vi "ChannelAutomatorR.vi"() -> ()   [LabVIEW 2020]
uses:
  <vilib>/Platform/TimedLoop/XDataNode/timing_clust.ctl
  <vilib>/Platform/TimedLoop/XDataNode/nitl_modes.ctl
  <vilib>/Platform/TimedLoop/XDataNode/wakeup.ctl
  bbe0dff6-800f-412b-80fa-b33fe90fb9f3.vi
  <vilib>/DAQmx/read.llb/DAQmx Read (Analog 1D Wfm NChan NSamp).vi
  <vilib>/DAQmx/write.llb/DAQmx Write (Analog 1D Wfm NChan NSamp).vi
  <vilib>/DAQmx/create/channels.llb/DAQmx Create Channel (AI-Voltage-Basic).vi
  <vilib>/httpClient/POSTBuffer.vi
  <vilib>/DAQmx/miscellaneous.llb/DAQmx Fill In Error Info.vi
  <vilib>/DAQmx/configure/timing.llb/DAQmx Timing (Sample Clock).vi
  <vilib>/DAQmx/create/channels.llb/DAQmx Create Channel (AO-Voltage-Basic).vi
  <vilib>/Comparison/Less/Less Functor/Less Functor.lvclass
  <vilib>/Platform/TimedLoop/XDataNode/XDataNode.xnode
  <resource>/objmgr/daqmx.rc
  <vilib>/httpClient/LabVIEWHTTPClient.lvlib
  <vilib>/wsapi/NI_WebServices.lvlib
  <vilib>/measure/NI_MABase.lvlib
  <vilib>/Platform/TimedLoop/XDataNode/XDNodeRunTimeDep.lvlib
  <vilib>/ptbypt/NI_PtbyPt.lvlib
panel:
  out "stds":dbl[](array[numeric])
  out "Means":dbl[](array[numeric])
  out "frequency":dbl=20.0
  out "fileCreateTime":timestamp
  out "headers":string
  out "timed out?":bool
  out "# elements in queue":i32
  out "body 2":string
  out "error out 3":errorcluster
  out "error out 2":errorcluster
  out "body":string
  in  "Tab Control 2":enum32{"RT Monitor", "IV Monitor"}(tab)
  out "Channel 4":waveform(dbl)[](graph)
  out "Channel 3":waveform(dbl)[](graph)
  out "Channel 2":waveform(dbl)[](graph)
  out "XY Graph":cluster{"Y":dbl[], "Y":dbl[]}[](graph)
  out "XY Graph 2":cluster{"Y":dbl[], "Y":dbl[]}[](graph)
  out "XY Graph 3":cluster{"Y":dbl[], "Y":dbl[]}[](graph)
  out "XY Graph 4":cluster{"Y":dbl[], "Y":dbl[]}[](graph)
  out "output path":path
  out "FilenameValid":bool
  out "ParameterNames":string[](array[string])=["Wafer", "Notes", "Experiment Name", "Buffer", "Bias Voltage", "Reference Electrode", "Chip", "Analyte"]
  out "ParameterValues":string[](array[string])
  out "RT Monitoring 2":bool
  out "error out":errorcluster
  out "StopProgram":bool
  out "FileOpen":bool
  out "tdms file out":refnum<k34>
  in  "Tab Control":enum32{"Data View", "Settings"}(tab)
  in  "TraceTime":dbl=30.0
  in  "IV Monitoring":bool
  in  "RT Monitoring":bool
  out "Recording":bool
  in  "Record":bool
  in  "Reference Voltage (mV)":string
  in  "Bias Voltage (mV)":string
  in  "Experiment Name":string
  in  "Wafer, Chip":string
  in  "Notes":string
  in  "Buffer":string
  in  "Analyte":string
  in  "DB48":bool
  in  "DB37":bool
  in  "Device Banks":bool
  in  "DB26":bool
  in  "Channels":string="N2,N6,E2,E6,S2,S6,W2,W6"
  out "Warnings":string="Wrong number of Channel Names!"
  out "Monitoring":bool
  in  "DataDirectory":path=path "C:/DempBot_Data"
  in  "Queue Size":i32=100
  in  "Channel 9":tag="Dev1/ai0"
  in  "Channel 10":tag="Dev1/ai2"
  in  "Channel 11":tag="Dev1/ai3"
  in  "Channel 12":tag="Dev1/ai4"
  in  "Channel 13":tag="Dev1/ai5"
  in  "Channel 14":tag="Dev1/ai6"
  in  "Channel 15":tag="Dev1/ai7"
  in  "Channel 16":tag="Dev1/ai8"
  in  "Sampling Rate:":dbl=5000.0
  in  "Recorded Channels":i32=8
  in  "No. of Samples / Loop":i64=1000
  in  "Gain (V/nA)":dbl=-0.45
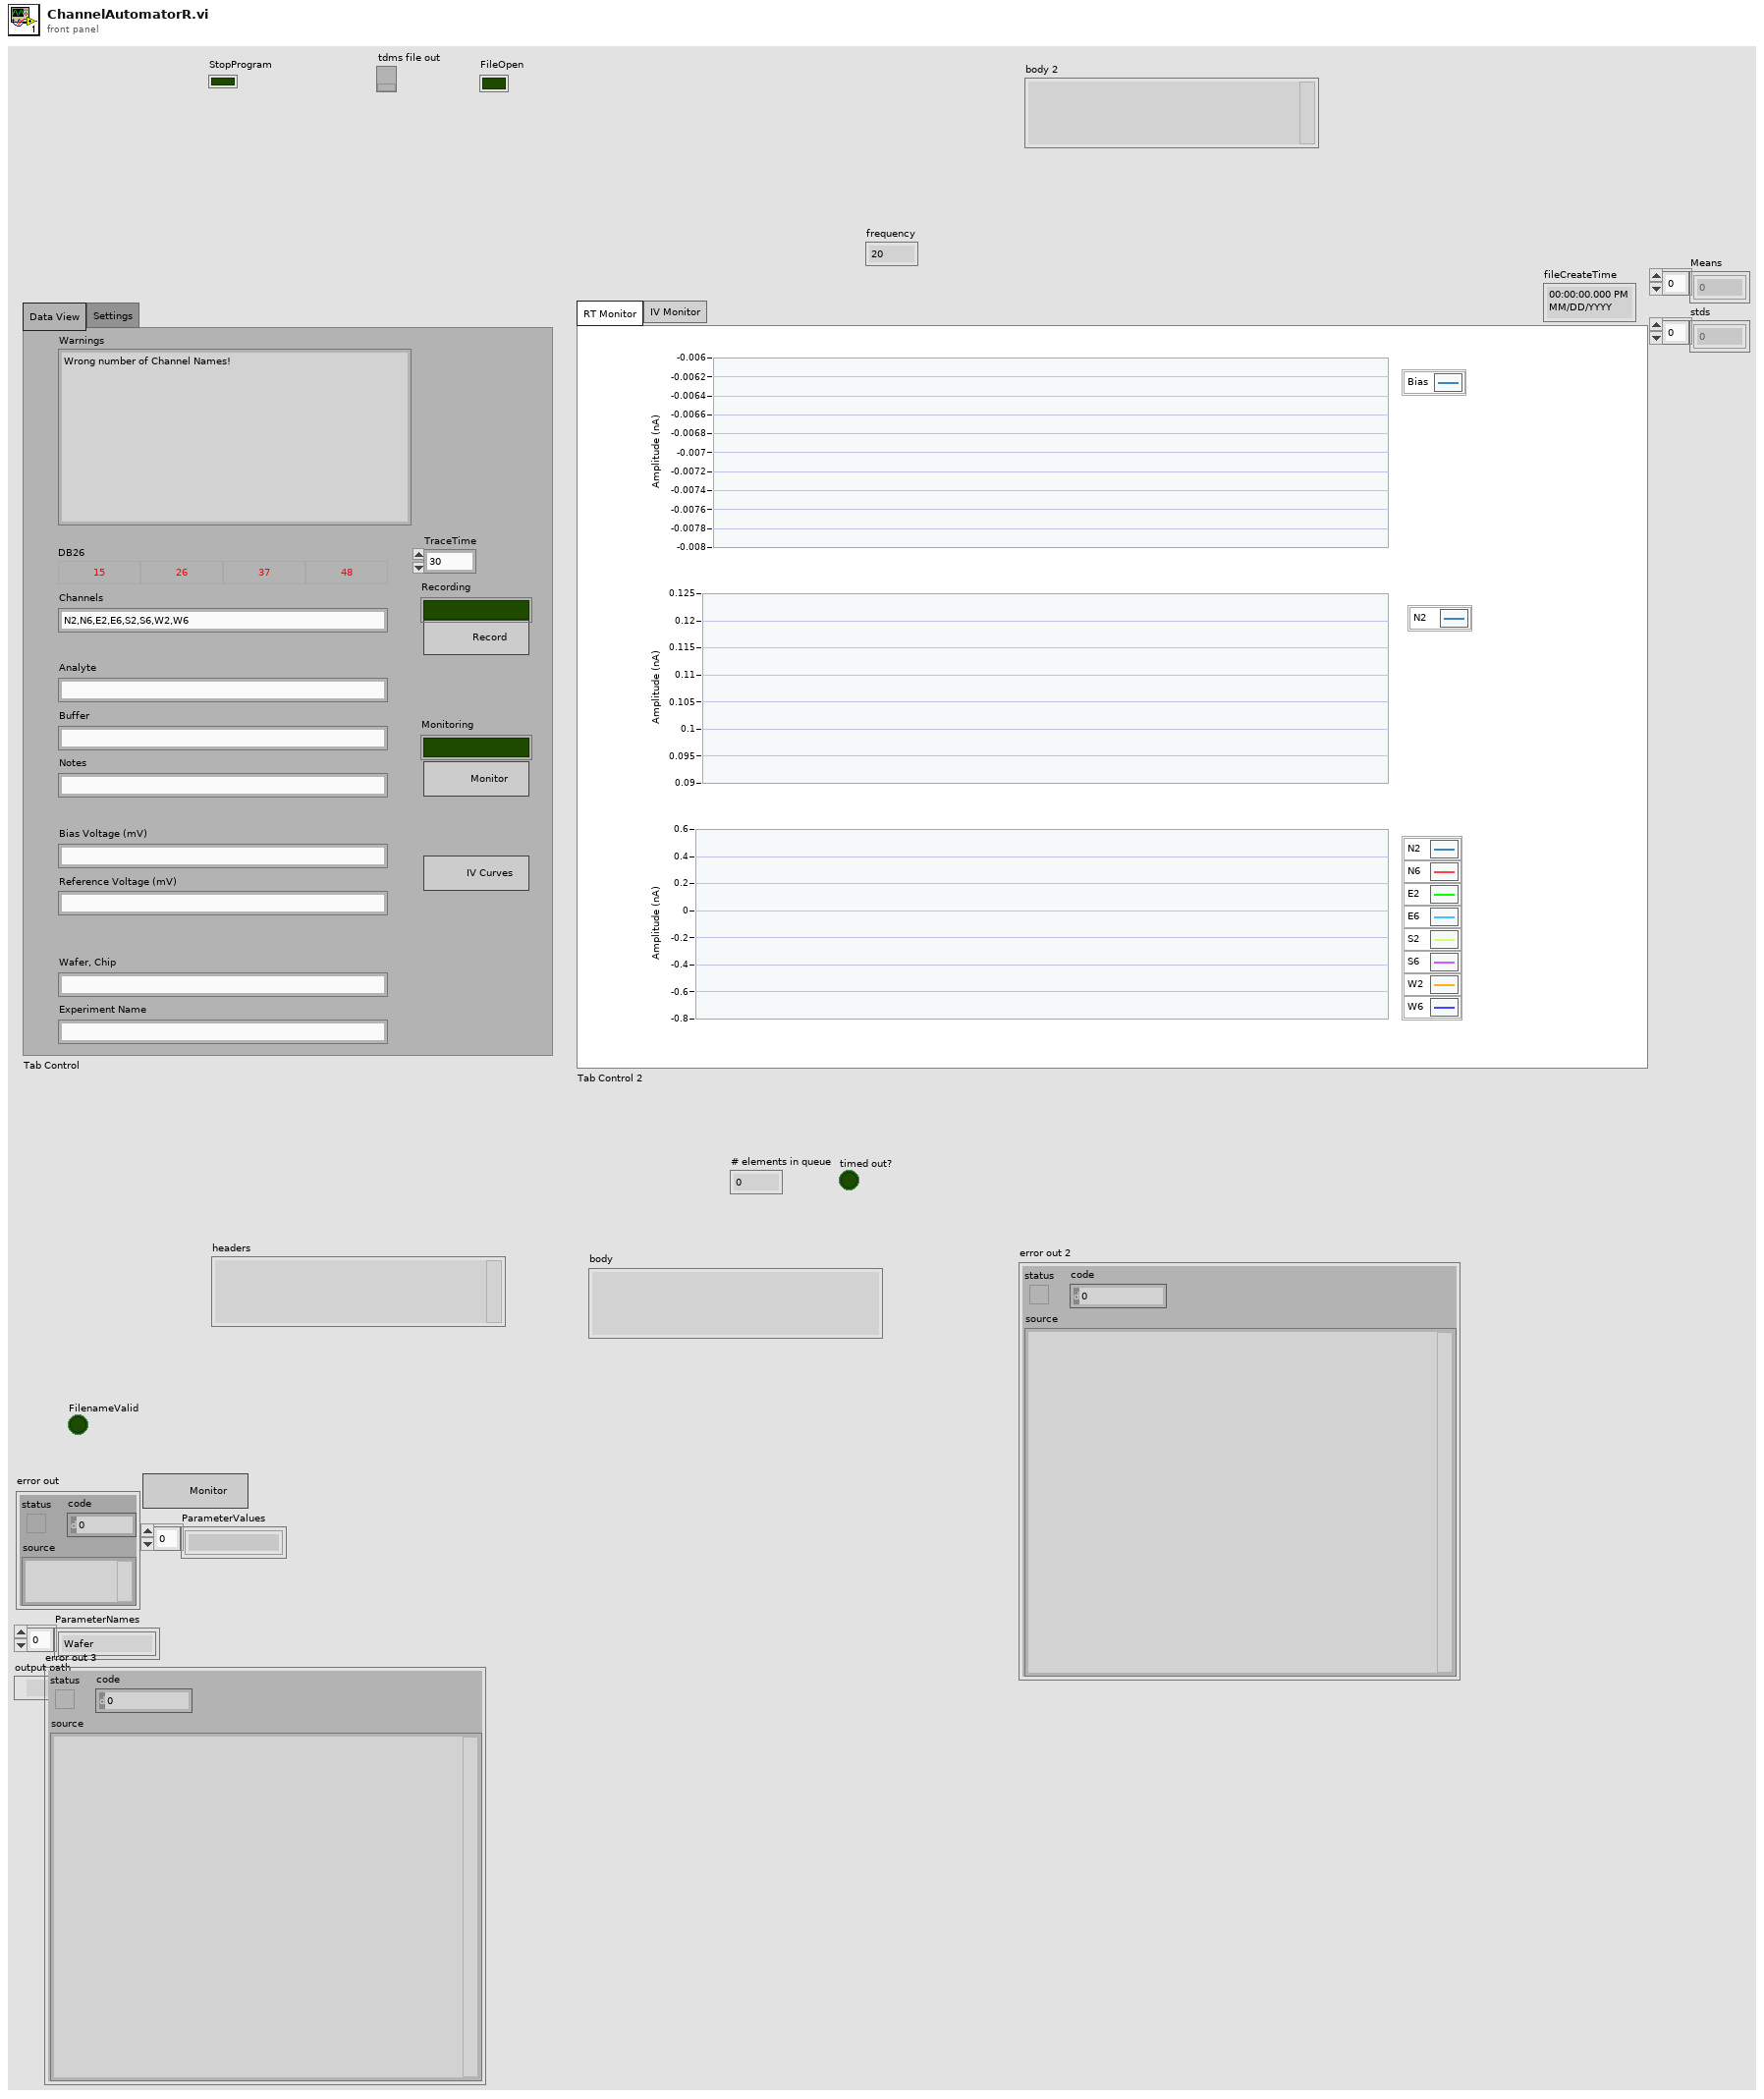
[diagram p1: front panel]
types:
  T1 = cluster{"command":string, "machine":string, "payload":string}
  T2 = typedef "LabVIEWHTTPClient.lvlib/ClientHandle.ctl" = refnum<k1>
  T3 = enum16{"open", "open or create", "create or replace", "create", "open (read-only)"}
  T4 = typedef "XDNodeRunTimeDep.lvlib/timing_clust.ctl" = cluster{"Expected End [f-1]":u64, "Actual End [f-1]":u64, "Finished Late? [f-1]":bool, "Expected End [i-1]":u64, "Actual End [i-1]":u64, "Finished Late? [i-1]":bool, "Expected Start [i]":u64, "Actual Start [i]":u64, "Expected Start [f]":u64, "Actual Start [f]":u64, "Source Name":string, "Structure Name":string, "Period":i64, "Deadline":i64, "Offset":i64, "Start":i64, "Priority":i32, "Timeout":i32, "Mode":T5, "Wakeup Reason":T6, "Error":errorcluster, "Source Type":string, "Secondary Source Type":string, "Global End Time":u64, "Global Start Time":u64, "Frame Duration":u64, "Iteration Duration":u64, "Assigned CPU":i32, "I/O Scan Engine Mode":u32}
  T5 = typedef "XDNodeRunTimeDep.lvlib/nitl_modes.ctl" = enum32{"No Change", "Process missed periods, maintain original phase", "Discard missed periods, maintain original phase", "Process missed periods, ignore original phase", "Discard missed periods, ignore original phase"}
  T6 = typedef "XDNodeRunTimeDep.lvlib/wakeup.ctl" = enum32{"Normal", "Aborted", "Asynchronous wakeup", "Timing source error", "Timed loop error", "Timeout"}
  T7 = enum16{"Sine Wave", "Triangle Wave", "Square Wave", "Sawtooth Wave"}
  T8 = cluster{"channelNames":string[], "dt":dbl, "traces":sgl[][], "dataType":string, "means":dbl[], "stds":dbl[]}
  T9 = cluster{"channels":string, "analyte":string, "notes":string, "buffer":string, "experiment":string, "waferChip":string}
  T10 = cluster{"duration":dbl, "bias":dbl, "frequency":dbl}
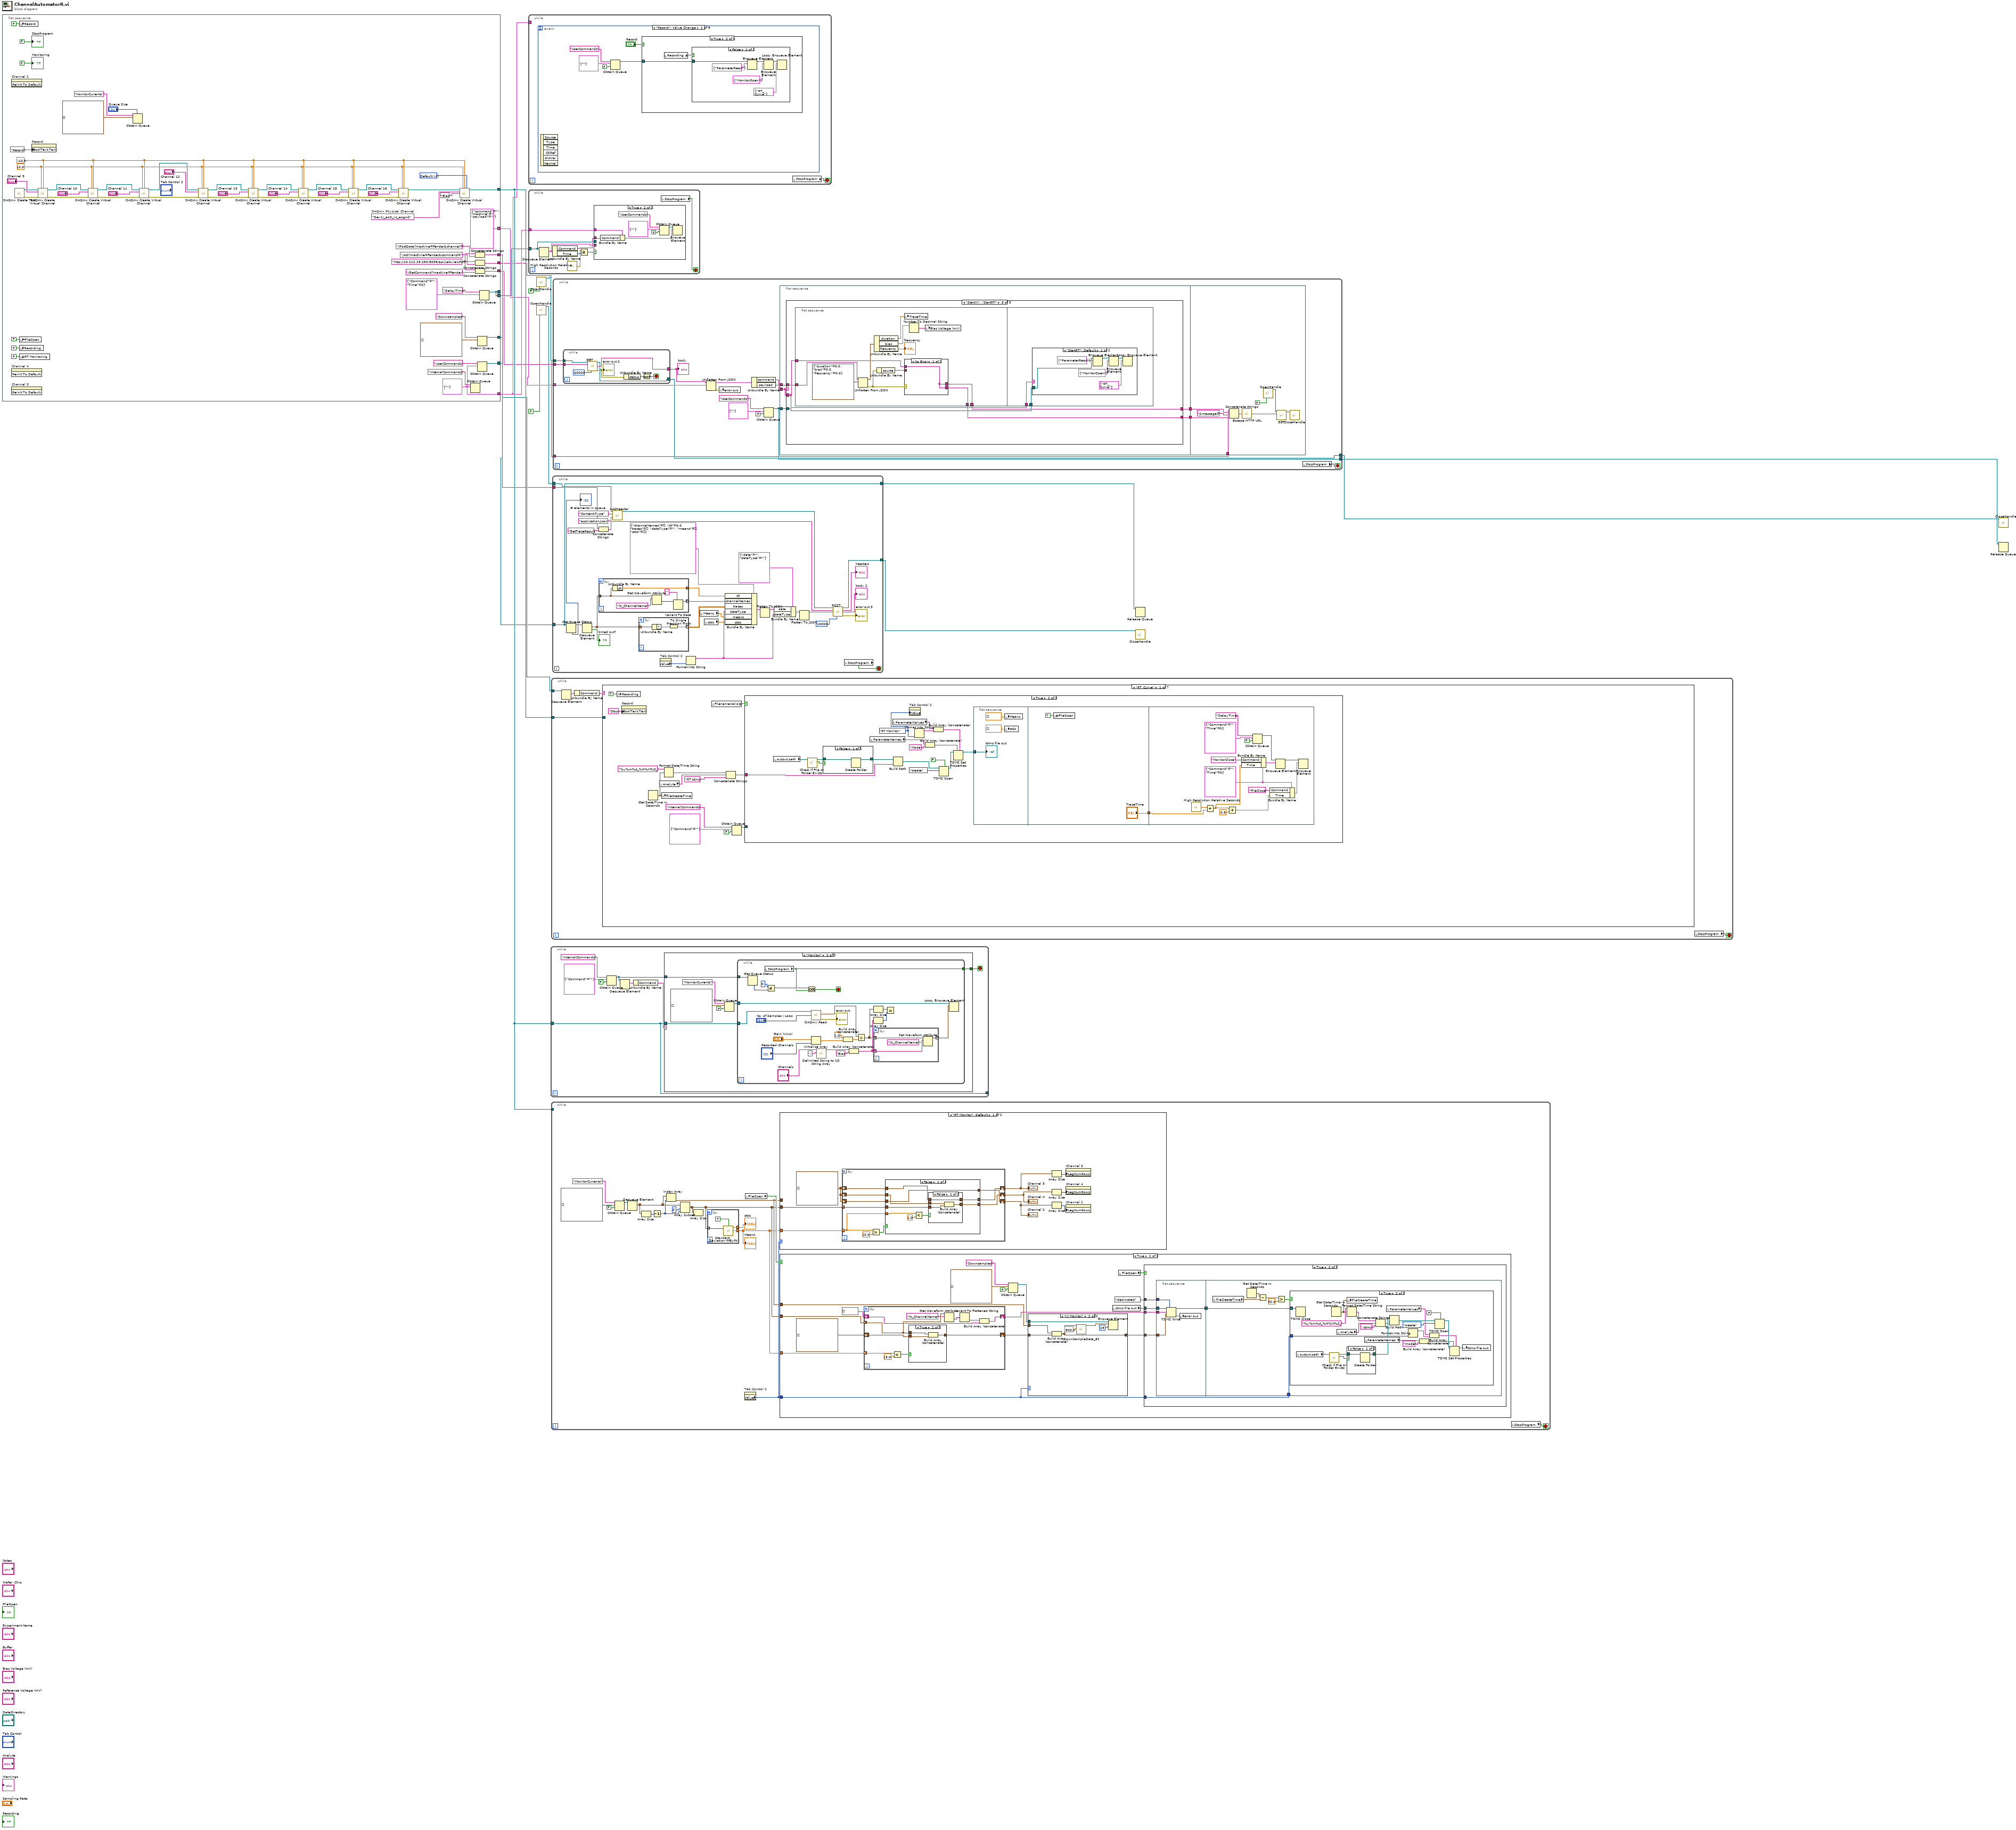
[diagram p0: block diagram]
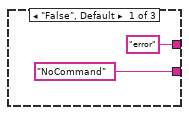
[diagram p2: hidden frame]
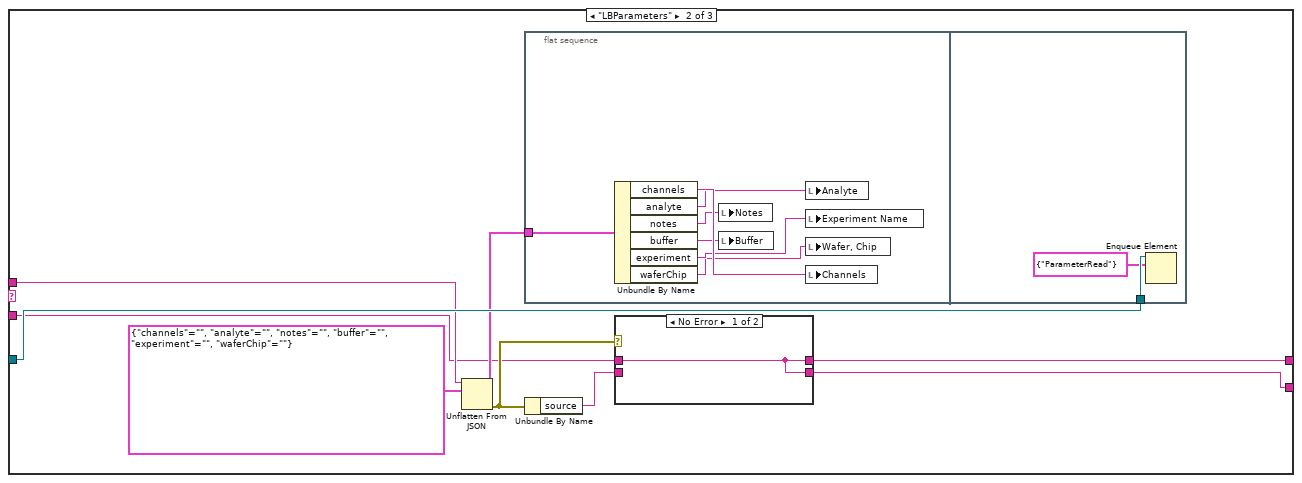
[diagram p3: hidden frame]
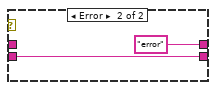
[diagram p4: hidden frame]
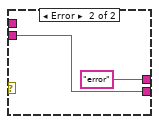
[diagram p5: hidden frame]
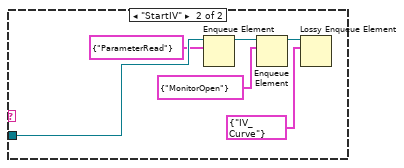
[diagram p6: hidden frame]
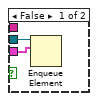
[diagram p7: hidden frame]
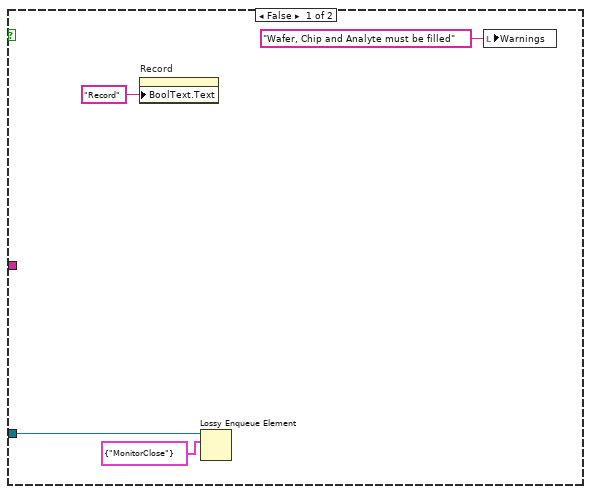
[diagram p8: hidden frame]
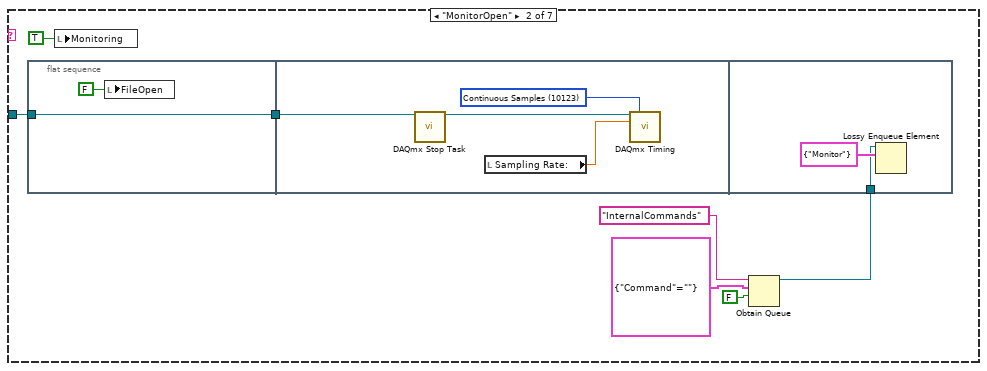
[diagram p10: hidden frame]
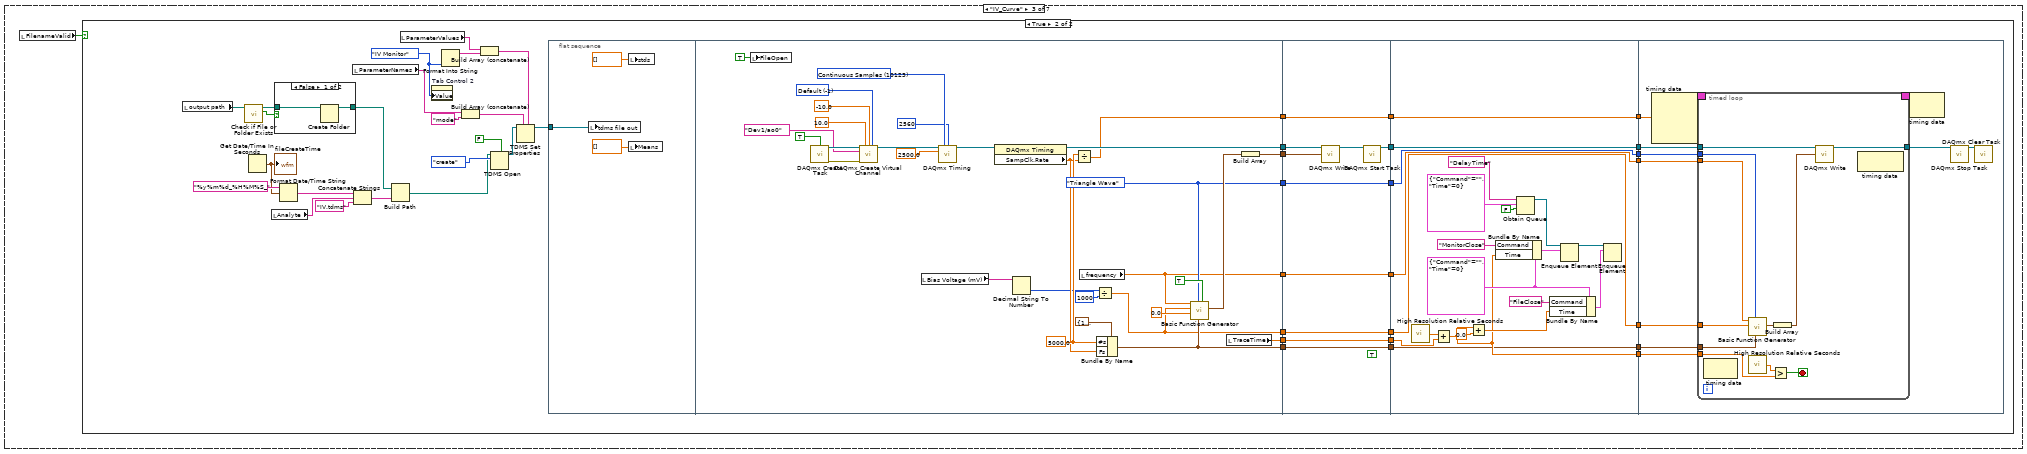
[diagram p11: hidden frame]
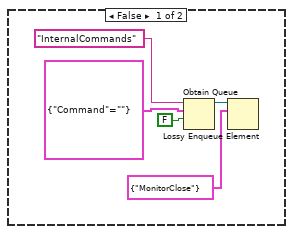
[diagram p12: hidden frame]
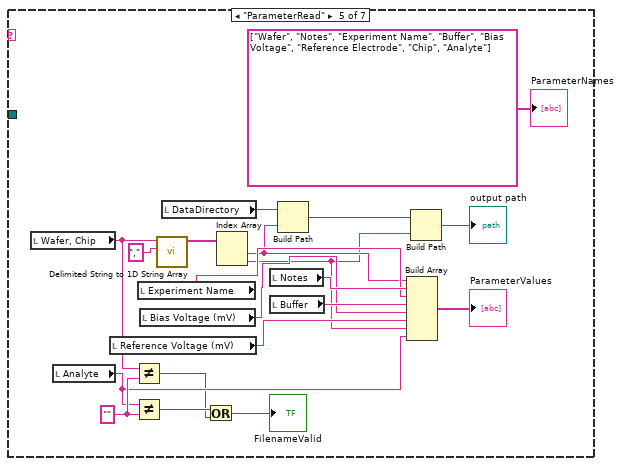
[diagram p15: hidden frame]
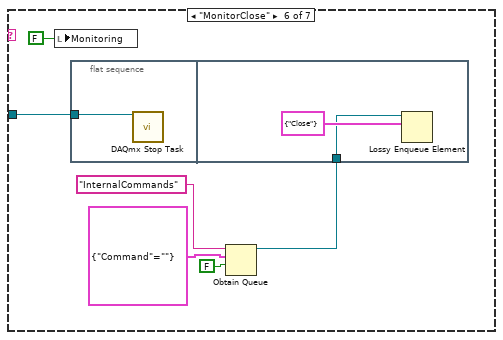
[diagram p16: hidden frame]
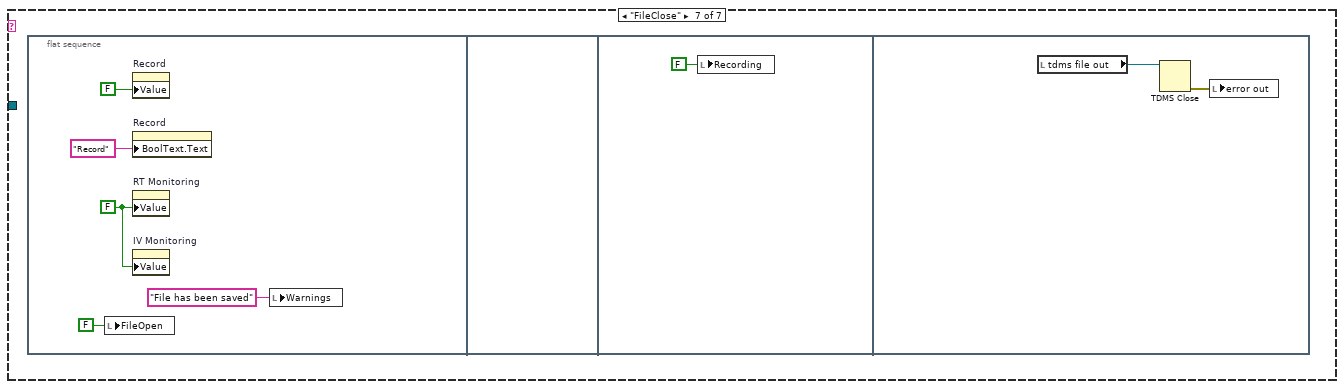
[diagram p17: hidden frame]
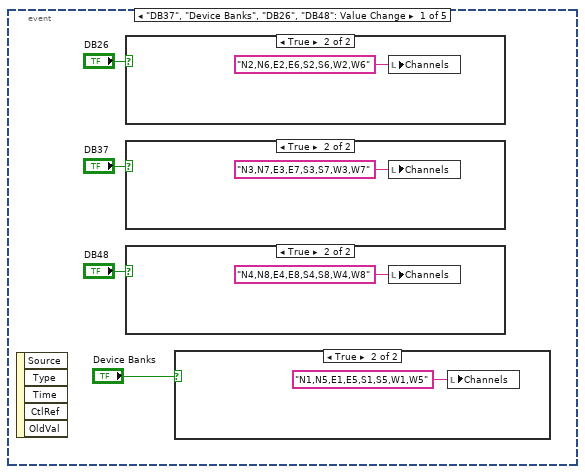
[diagram p18: hidden frame]
diagram:
  n1 = flat-sequence {
    tunnel: [w35] -> w17
    tunnel: [w40] -> w15
    tunnel: [w30] -> w16
    tunnel: [w34] -> w14
    tunnel: [w30] -> _
    tunnel: [T1 {"command"="", "machine"="", "payload"=""}] -> w13
    tunnel: [w28] -> w12
    tunnel: [w23] -> w9
    tunnel: [w22] -> w8
    tunnel: [w24] -> w1
    frame #0 {
      w20 = -1 items=["Default"=-1, "RSE"=10083, "NRSE"=10078, "Differential"=10106, "Pseudodifferential"=12529] ("input terminal configuration")
      w21 = "http://10.212.29.250:8038/api/LabviewPoll"
      w42 = tag "Dev1/_ao0_vs_aognd"  # DAQmx Physical Channel
      w34 = cluster{"Command":string} {"Command"=""}
      w19 = -10.0 ("minimum value")
      w18 = 10.0 ("maximum value")
      n2 = invoke on="Channel 2" class="WFChart (strict)" method="Reinit To Default"() -> ()  [unwired: 3 in, 3 out]
      n3 = invoke on="Channel 4" class="WFChart (strict)" method="Reinit To Default"() -> ()  [unwired: 3 in, 3 out]
      n4 = invoke on="Channel 3" class="WFChart (strict)" method="Reinit To Default"() -> ()  [unwired: 3 in, 3 out]
      n5 = call <vilib>:"DAQmx Create Task.vi"() -> ("task out"=w54:refnum<k21>, "error out"=w53:errorcluster)  [unwired: 14 in]
      n6 = local write "Record"(FALSE ("Record")) -> ()
      n7 = local write "FileOpen"(FALSE ("FileOpen")) -> ()
      n8 = local write "Recording"(FALSE ("Recording")) -> ()
      n9 = local write "RT Monitoring"(FALSE ("RT Monitoring")) -> ()
      n10 = property on="Record" class="Bool (strict)"("BoolText.Text"="Record" ("Boolean Text.Text")) -> ()  [unwired: 2 in, 2 out]
      n11 = call-poly <vilib>:"DAQmx Create Virtual Channel.vi"("task in"=w54, "maximum value"=w18, "minimum value"=w19, "physical channels"="Channel 9", "error in"=w53) -> ("task out"=w76:refnum<k21>, "error out"=w69:errorcluster)  [unwired: 9 in]
      n12 = call-poly <vilib>:"DAQmx Create Virtual Channel.vi"("task in"=w76, "maximum value"=w18, "minimum value"=w19, "physical channels"="Channel 10", "error in"=w69) -> ("task out"=w75:refnum<k21>, "error out"=w68:errorcluster)  [unwired: 9 in]
      n13 = Obtain Queue(max queue size (-1, unlimited)="Queue Size", name (unnamed)="MonitorCurrents", element data type=waveform(dbl)[] []) -> ()  [unwired: 2 in, 3 out]
      n14 = call-poly <vilib>:"DAQmx Create Virtual Channel.vi"("task in"=w75, "maximum value"=w18, "minimum value"=w19, "physical channels"="Channel 11", "error in"=w68) -> ("task out"=w74:refnum<k21>, "error out"=w67:errorcluster)  [unwired: 9 in]
      n15 = call-poly <vilib>:"DAQmx Create Virtual Channel.vi"("task in"=w74, "maximum value"=w18, "minimum value"=w19, "physical channels"="Channel 12", "error in"=w67) -> ("task out"=w66:refnum<k21>, "error out"=w65:errorcluster)  [unwired: 9 in]
      n16 = call-poly <vilib>:"DAQmx Create Virtual Channel.vi"("task in"=w66, "maximum value"=w18, "minimum value"=w19, "physical channels"="Channel 13", "error in"=w65) -> ("task out"=w63:refnum<k21>, "error out"=w62:errorcluster)  [unwired: 9 in]
      n17 = call-poly <vilib>:"DAQmx Create Virtual Channel.vi"("task in"=w63, "maximum value"=w18, "minimum value"=w19, "physical channels"="Channel 14", "error in"=w62) -> ("task out"=w61:refnum<k21>, "error out"=w60:errorcluster)  [unwired: 9 in]
      n18 = call-poly <vilib>:"DAQmx Create Virtual Channel.vi"("task in"=w61, "maximum value"=w18, "minimum value"=w19, "physical channels"="Channel 15", "error in"=w60) -> ("task out"=w59:refnum<k21>, "error out"=w58:errorcluster)  [unwired: 9 in]
      n19 = call-poly <vilib>:"DAQmx Create Virtual Channel.vi"("task in"=w59, "maximum value"=w18, "minimum value"=w19, "physical channels"="Channel 16", "error in"=w58) -> ("task out"=w41:refnum<k21>)  [unwired: 9 in, 1 out]
      n20 = call-poly <vilib>:"DAQmx Create Virtual Channel.vi"("task in"=w41, "maximum value"=w18, "minimum value"=w19, "input terminal configuration"=w20, "physical channels"=w42, "name to assign"="Bias") -> ("task out"=w40:refnum<k21>)  [unwired: 8 in, 1 out]
      n21 = Obtain Queue(name (unnamed)="InternalCommands", element data type=w34) -> ()  [unwired: 3 in, 3 out]
      n22 = Concatenate Strings(w21, "/PostData?machine=Fender&channel=" ("url")) -> (w22:string)
      n23 = Concatenate Strings(w21, "/Ack?machine=Fender&command=" ("url")) -> (w24:string)
      n24 = Concatenate Strings(w21, "/GetCommand?machine=Fender" ("url")) -> (w23:string)
      n25 = Obtain Queue(name (unnamed)="Downsampled", element data type=waveform(dbl)[] []) -> (queue out=w28:refnum<queue>)  [unwired: 3 in, 2 out]
      n26 = Obtain Queue(name (unnamed)="UserCommands", element data type=w34) -> (queue out=w35:refnum<queue>)  [unwired: 3 in, 2 out]
      n27 = Obtain Queue(name (unnamed)="DelayTime", element data type=cluster{"Command":string, "Time":i32} {"Command"="", "Time"=0}) -> (queue out=w30:refnum<queue>)  [unwired: 3 in, 2 out]
      "StopProgram" <- FALSE ("StopProgram")
      "Monitoring" <- FALSE ("Monitoring")
    }
  }
  n28 = while {
    tunnel: w14 -> [_]
    stop <- w77 stop-if-true
    n29 = event shown="[1] \"Record\": Value Change" {
      selector: _ -> [_ _ _ _ _]
      dyn-events: _ -> [_ _ _ _ _]
      timeout: _ -> [_ _ _ _ _]
      event "DB37", "Device Banks", "DB26", "DB48": Value Change {
        n30 = event-data() -> ()  [unwired: 1 in, 5 out]
        n31 = case shown="True" "DB26" {
          frame False {
          }
          frame True {
            n32 = local write "Channels"("N2,N6,E2,E6,S2,S6,W2,W6" ("Channels")) -> ()
          }
        }
        n33 = case shown="True" "DB37" {
          frame False {
          }
          frame True {
            n34 = local write "Channels"("N3,N7,E3,E7,S3,S7,W3,W7" ("Channels")) -> ()
          }
        }
        n35 = case shown="True" "DB48" {
          frame False {
          }
          frame True {
            n36 = local write "Channels"("N4,N8,E4,E8,S4,S8,W4,W8" ("Channels")) -> ()
          }
        }
        n37 = case shown="True" "Device Banks" {
          frame False {
          }
          frame True {
            n38 = local write "Channels"("N1,N5,E1,E5,S1,S5,W1,W5" ("Channels")) -> ()
          }
        }
      }
      event "Record": Value Change {
        n39 = event-data() -> ()  [unwired: 1 in, 6 out]
        n40 = Obtain Queue(name (unnamed)="UserCommands", element data type=cluster{"Command":string} {"Command"=""}, create if not found? (T)=FALSE) -> (queue out=w86:refnum<queue>)  [unwired: 2 in, 2 out]
        n41 = case shown="True" "Record" {
          tunnel: w86 -> [w91 w95]
          frame False {
            n42 = Enqueue Element(queue=w91, element=cluster{"Command":string} {"Command"="MonitorClose"}) -> (queue out=w93:refnum<queue>)  [unwired: 2 in, 2 out]
            n43 = Lossy Enqueue Element(queue=w93, element=cluster{"Command":string} {"Command"="File_Close"}) -> ()  [unwired: 1 in, 4 out]
          }
          frame True {
            n44 = local read "Recording"() -> (w96:bool)
            n45 = case shown="False" w96 {
              tunnel: w95 -> [w99 w103]
              frame False {
                n46 = Enqueue Element(queue=w99, element=cluster{"Command":string} {"Command"="ParameterRead"}) -> (queue out=w97:refnum<queue>)  [unwired: 2 in, 2 out]
                n47 = Enqueue Element(queue=w97, element=cluster{"Command":string} {"Command"="MonitorOpen"}) -> (queue out=w101:refnum<queue>)  [unwired: 2 in, 2 out]
                n48 = Lossy Enqueue Element(queue=w101, element=cluster{"Command":string} {"Command"="RT_Curve"}) -> ()  [unwired: 1 in, 4 out]
              }
              frame True {
                n49 = Lossy Enqueue Element(queue=w103, element=cluster{"Command":string} {"Command"="FileClose"}) -> ()  [unwired: 1 in, 4 out]
              }
            }
          }
        }
      }
      event "IV Monitoring": Value Change {
        n50 = event-data() -> ()  [unwired: 1 in, 6 out]
        n51 = Obtain Queue(name (unnamed)="UserCommands", element data type=cluster{"Command":string} {"Command"=""}, create if not found? (T)=FALSE) -> (queue out=w106:refnum<queue>)  [unwired: 2 in, 2 out]
        n52 = Enqueue Element(queue=w106, element=cluster{"Command":string} {"Command"="ParameterRead"}) -> (queue out=w105:refnum<queue>)  [unwired: 2 in, 2 out]
        n53 = Enqueue Element(queue=w105, element=cluster{"Command":string} {"Command"="MonitorOpen"}) -> (queue out=w111:refnum<queue>)  [unwired: 2 in, 2 out]
        n54 = Lossy Enqueue Element(queue=w111, element=cluster{"Command":string} {"Command"="IV_Curve"}) -> ()  [unwired: 1 in, 4 out]
      }
      event "RT Monitoring": Value Change {
        n55 = event-data() -> ()  [unwired: 1 in, 6 out]
        n56 = local read "Monitoring"() -> (w119:bool)
        n57 = Obtain Queue(name (unnamed)="UserCommands", element data type=cluster{"Command":string} {"Command"=""}, create if not found? (T)=FALSE) -> (queue out=w114:refnum<queue>)  [unwired: 2 in, 2 out]
        n58 = case shown="False" w119 {
          tunnel: w114 -> [w120 w123]
          frame False {
            n59 = Lossy Enqueue Element(queue=w120, element=cluster{"Command":string} {"Command"="MonitorOpen"}) -> ()  [unwired: 1 in, 4 out]
          }
          frame True {
            n60 = Lossy Enqueue Element(queue=w123, element=cluster{"Command":string} {"Command"="MonitorClose"}) -> ()  [unwired: 1 in, 4 out]
          }
        }
        "RT Monitoring 2" <- "RT Monitoring"
      }
      event "Wafer, Chip", "Experiment Name", "Bias Voltage (mV)", "Reference Voltage (mV)", "Notes", "Buffer", "Analyte": Value Change {
        n61 = event-data() -> ()  [unwired: 1 in, 6 out]
        n62 = Obtain Queue(name (unnamed)="UserCommands", element data type=cluster{"Command":string} {"Command"=""}, create if not found? (T)=FALSE) -> (queue out=w124:refnum<queue>)  [unwired: 2 in, 2 out]
        n63 = Enqueue Element(queue=w124, element=cluster{"Command":string} {"Command"="ParameterRead"}) -> ()  [unwired: 2 in, 3 out]
      }
    }
    n64 = local read "StopProgram"() -> (w77:bool)
  }
  n65 = while {
    tunnel: w16 -> [w134]
    tunnel: w14 -> [w135]
    stop <- w133 stop-if-true
    n66 = Dequeue Element(queue=w134) -> (element=w136:cluster{"Command":string, "Time":i32})  [unwired: 2 in, 3 out]
    n67 = Unbundle By Name(w136) -> ("Command"=w129:string, "Time"=w132:i32)
    n68 = call <vilib>:"High Resolution Relative Seconds.vi"() -> ("relative seconds"=w131:dbl)
    n69 = Greater Or Equal?(x=w131, y=w132) -> (x >= y?=w130:bool)
    n70 = case shown="True" w130 {
      tunnel: w135 -> [_ w145]
      tunnel: w129 -> [_ w144]
      tunnel: w134 -> [w138 _]
      tunnel: w136 -> [w137 _]
      frame False {
        n71 = Enqueue Element(queue=w138, element=w137) -> ()  [unwired: 2 in, 3 out]
      }
      frame True {
        n72 = Bundle By Name(cluster=w145, "Command"=w144) -> (w143:cluster{"Command":string})
        n73 = Obtain Queue(name (unnamed)="UserCommands", element data type=cluster{"Command":string} {"Command"=""}, create if not found? (T)=FALSE) -> (queue out=w139:refnum<queue>)  [unwired: 2 in, 2 out]
        n74 = Enqueue Element(queue=w139, element=w143) -> ()  [unwired: 2 in, 3 out]
      }
    }
    n75 = local read "StopProgram"() -> (w133:bool)
  }
  n76 = call <vilib>:"OpenHandle.vi"("verify server(true)"=FALSE) -> ("client handle out"=w3:T2)  [unwired: 13 in, 1 out]
  n77 = call <vilib>:"OpenHandle.vi"("verify server(true)"=FALSE) -> ("client handle out"=w6:T2)  [unwired: 13 in, 1 out]
  n78 = while {
    tunnel: [w152] -> _
    tunnel: w15 -> [w152]
    stop <- w153 stop-if-true
    n79 = Obtain Queue(name (unnamed)="InternalCommands", element data type=cluster{"Command":string} {"Command"=""}, create if not found? (T)=FALSE) -> (queue out=w147:refnum<queue>)  [unwired: 2 in, 2 out]
    n80 = Dequeue Element(queue=w147) -> (element=w151:cluster{"Command":string})  [unwired: 2 in, 3 out]
    n81 = Unbundle By Name(w151) -> ("Command"=w150:string)
    n82 = case shown="\"Monitor\"" w150 {
      tunnel: [w154 w161] -> w153
      tunnel: w152 -> [_ w160]
      tunnel: w147 -> [_ w159]
      frame "False", Default {
        n83 = local read "StopProgram"() -> (w154:bool)
      }
      frame "Monitor" {
        n84 = Obtain Queue(name (unnamed)="MonitorCurrents", element data type=waveform(dbl)[] [], create if not found? (T)=FALSE) -> (queue out=w155:refnum<queue>)  [unwired: 2 in, 2 out]
        n85 = while {
          tunnel: w155 -> [w179]
          tunnel: [w167] -> w161
          tunnel: w160 -> [w172]
          tunnel: w159 -> [w171]
          stop <- w168 stop-if-true
          n86 = Get Queue Status(queue=w171) -> (# elements in queue=w170:i32)  [unwired: 2 in, 7 out]
          n87 = local read "StopProgram"() -> (w167:bool)
          n88 = Not Equal?(x=0, y=w170) -> (x != y?=w169:bool)
          n89 = Or(x=w169, y=w167) -> (x .or. y?=w168:bool)
          n90 = call-poly <vilib>:"DAQmx Read.vi"("task/channels in"=w172, "number of samples per channel"="No. of Samples / Loop") -> ("data"=w180:waveform(dbl)[], "error out"=→"error out":errorcluster)  [unwired: 11 in, 1 out]
          n91 = Initialize Array("Gain (V/nA)", "Recorded Channels") -> (w183:dbl[])
          n92 = call <vilib>:"Delimited String to 1D String Array.vi"("delimiter"="," ("search string/char (-)"), "delimited string"="Channels") -> ("string array"=w164:string[])  [unwired: 9 in]
          n93 = Build Array (concatenate)(1.0 ("Gain (V/nA)"), w183) -> (w181:dbl[])
          n94 = Build Array (concatenate)(w164, "Bias") -> (w163:string[])
          n95 = Divide(x=w180, y=w181) -> (x/y=w175:waveform(dbl)[])
          n96 = Array Size(array=w175) -> (size(s)=w174:i32)
          n97 = Array Size(array=w163) -> (size(s)=w173:i32)
          n98 = for {
            tunnel: w175 -> [w190] mode=indexing
            tunnel: w163 -> [w188] mode=indexing
            tunnel: [w187] -> w176 mode=indexing
            n99 = Set Waveform Attribute(5:w188, 6:"NI_ChannelName" ("name"), 7:w190) -> (3:w187:waveform(dbl))  [unwired: 1 in, 2 out]
          }
          n100 = Equal?(x=w174, y=w173) -> ()  [unwired: 1 out]
          n101 = Lossy Enqueue Element(queue=w179, element=w176) -> ()  [unwired: 1 in, 4 out]
        }
      }
    }
  }
  n102 = while {
    tunnel: w15 -> [_]
    stop <- w205 stop-if-true
    n103 = Obtain Queue(name (unnamed)="MonitorCurrents", element data type=waveform(dbl)[] [], create if not found? (T)=FALSE) -> (queue out=w198:refnum<queue>)  [unwired: 2 in, 2 out]
    n104 = Dequeue Element(queue=w198) -> (element=w193:waveform(dbl)[])  [unwired: 2 in, 3 out]
    n105 = Array Size(array=w193) -> (size(s)=w203:i32)
    n106 = Decrement(x=w203) -> (x-1=w202:i32)
    n107 = Index Array(array=w193, index=w202) -> (element=w196:waveform(dbl))
    n108 = Array Subset(array=w193, index=0, length=w202) -> (w195:waveform(dbl)[])
    n109 = Array Size(array=w195) -> ()  [unwired: 1 out]
    n110 = for {
      tunnel: w195 -> [w409] mode=indexing
      tunnel: [w407] -> w191 mode=indexing
      tunnel: [w406] -> w192 mode=indexing
      n111 = call <vilib>:"Standard Deviation PtByPt.vi"("x"=w409, "initialize"=TRUE) -> ("standard deviation"=w407:dbl, "mean"=w406:dbl)  [unwired: 1 in, 1 out]
    }
    "Means" <- w192
    "stds" <- w191
    n112 = property on="Tab Control 2" class="TabCtl (strict)"() -> ("Value"=w197:enum32{"RT Monitor", "IV Monitor"})  [unwired: 2 in, 2 out]
    n113 = local read "FileOpen"() -> (w204:bool)
    n114 = case shown="\"RT Monitor\", Default" w197 {
      tunnel: w195 -> [w206 w248]
      tunnel: w192 -> [w207 _]
      tunnel: w196 -> [_ w261]
      frame "RT Monitor", Default {
        w208 = waveform(dbl)[] []
        n115 = for {
          tunnel: w206 -> [w223] mode=indexing
          tunnel: w207 -> [w220] mode=indexing
          shift-right: [w222] -> w209
          shift-left: w208 -> [w221]
          shift-right: [w219] -> w214
          shift-left: w208 -> [w218]
          shift-right: [w217] -> w211
          shift-left: w208 -> [w216]
          n116 = Greater?(x=w220, y=10.0) -> (0:w224:bool)
          n117 = case shown="False" w224 {
            tunnel: w223 -> [w230 w246]
            tunnel: [w233 w245] -> w222
            tunnel: w221 -> [w233 w244]
            tunnel: w220 -> [w232 _]
            tunnel: [w229 w243] -> w219
            tunnel: w218 -> [w228 w243]
            tunnel: [w227 w242] -> w217
            tunnel: w216 -> [w226 w242]
            frame False {
              n118 = Less?(x=w232, y=1.0) -> (x < y?=w231:bool)
              n119 = case shown="False" w231 {
                tunnel: w230 -> [w236 w241]
                tunnel: [w237 w240] -> w229
                tunnel: w228 -> [w237 w239]
                tunnel: [w235 w238] -> w227
                tunnel: w226 -> [w234 w238]
                frame False {
                  n120 = Build Array (concatenate)(w234, w236) -> (w235:waveform(dbl)[])
                }
                frame True {
                  n121 = Build Array (concatenate)(w239, w241) -> (w240:waveform(dbl)[])
                }
              }
            }
            frame True {
              n122 = Build Array (concatenate)(w244, w246) -> (w245:waveform(dbl)[])
            }
          }
        }
        "Channel 2" <- w209
        "Channel 3" <- w214
        "Channel 4" <- w211
        n123 = Array Size(array=w214) -> (size(s)=w213:i32)
        n124 = Array Size(array=w211) -> (size(s)=w212:i32)
        n125 = Array Size(array=w209) -> (size(s)=w210:i32)
        n126 = property on="Channel 3" class="WFChart (strict)"("LegNumRows"=w213) -> ()  [unwired: 2 in, 2 out]
        n127 = property on="Channel 4" class="WFChart (strict)"("LegNumRows"=w212) -> ()  [unwired: 2 in, 2 out]
        n128 = property on="Channel 2" class="WFChart (strict)"("LegNumRows"=w210) -> ()  [unwired: 2 in, 2 out]
      }
      frame "IV Monitor" {
        n129 = Unbundle By Name(w261) -> ("Y"=w255:dbl[])
        n130 = Array Size(array=w248) -> (size(s)=w247:i32)
        n131 = Array Max & Min(array=w255) -> (max value=w251:dbl)  [unwired: 3 out]
        n132 = for {
          tunnel: w248 -> [w268] mode=indexing
          tunnel: w251 -> [w266]
          tunnel: [w262] -> w250 mode=indexing
          n133 = Unbundle By Name(w268) -> ("Y"=w263:dbl[])
          n134 = Array Max & Min(array=w263) -> (max value=w267:dbl)  [unwired: 3 out]
          n135 = Divide(x=w267, y=w266) -> (x/y=w265:dbl)
          n136 = To Word Integer(number=w265) -> (16bit integer=w264:i16)
          n137 = Bundle(w264, "Y"=w263) -> (w262:cluster{i16, "Y":dbl[]})  [unwired: 1 in]
        }
        n138 = call "Sort 1D Array.vim"("unsorted array"=w250) -> ("sorted array"=w249:cluster{i16, "Y":dbl[]}[])  [unwired: 10 in]
        n139 = for {
          tunnel: w248 -> [_] mode=indexing
          shift-right: [w279] -> w252
          shift-left: cluster{"Y":dbl[], "Y":dbl[]}[] [] -> [w278]
          shift-right: [w282] -> w253
          shift-left: cluster{"Y":dbl[], "Y":dbl[]}[] [] -> [w283]
          shift-right: [w281] -> w256
          shift-left: cluster{"Y":dbl[], "Y":dbl[]}[] [] -> [w280]
          shift-right: [w284] -> w254
          shift-left: cluster{"Y":dbl[], "Y":dbl[]}[] [] -> [w285]
          tunnel: w255 -> [w277]
          tunnel: w251 -> [_]
          tunnel: w249 -> [w276] mode=indexing
          tunnel: w247 -> [w272]
          i -> [w274]
          n140 = Divide(x=w274, y=w272) -> (x/y=w273:dbl)
          n141 = Multiply(x=w273, y=8.0) -> (x*y=w271:dbl)
          n142 = Unbundle(w276) -> ("Y"=w275:dbl[])  [unwired: 1 out]
          n143 = To Long Integer(number=w271) -> (32bit integer=w269:i32)
          n144 = case shown="0, 1" w269 {
            tunnel: w285 -> [w290 w299 w304 w312]
            tunnel: w277 -> [w293 w296 w308 w316]
            tunnel: w275 -> [w292 w295 w307 w315]
            tunnel: [w289 w299 w304 w312] -> w284
            tunnel: w283 -> [w288 w298 w306 w311]
            tunnel: [w288 w298 w305 w311] -> w282
            tunnel: [w287 w300 w303 w310] -> w281
            tunnel: w280 -> [w287 w297 w303 w310]
            tunnel: [w286 w294 w302 w313] -> w279
            tunnel: w278 -> [w286 w294 w302 w314]
            frame 0, 1 {
              n145 = Bundle("Y"=w293, "Y"=w292) -> (w291:cluster{"Y":dbl[], "Y":dbl[]})  [unwired: 1 in]
              n146 = Build Array (concatenate)(w290, w291) -> (w289:cluster{"Y":dbl[], "Y":dbl[]}[])
            }
            frame 4, 5 {
              n147 = Bundle("Y"=w296, "Y"=w295) -> (w301:cluster{"Y":dbl[], "Y":dbl[]})  [unwired: 1 in]
              n148 = Build Array (concatenate)(w297, w301) -> (w300:cluster{"Y":dbl[], "Y":dbl[]}[])
            }
            frame 2, 3 {
              n149 = Bundle("Y"=w308, "Y"=w307) -> (w309:cluster{"Y":dbl[], "Y":dbl[]})  [unwired: 1 in]
              n150 = Build Array (concatenate)(w306, w309) -> (w305:cluster{"Y":dbl[], "Y":dbl[]}[])
            }
            frame 6, 7, Default {
              n151 = Bundle("Y"=w316, "Y"=w315) -> (w317:cluster{"Y":dbl[], "Y":dbl[]})  [unwired: 1 in]
              n152 = Build Array (concatenate)(w314, w317) -> (w313:cluster{"Y":dbl[], "Y":dbl[]}[])
            }
          }
        }
        "XY Graph" <- w254
        "XY Graph 2" <- w253
        "XY Graph 3" <- w256
        "XY Graph 4" <- w252
      }
    }
    n153 = case shown="True" w204 {
      tunnel: w195 -> [_ w333]
      tunnel: w192 -> [_ w332]
      tunnel: w196 -> [_ w328]
      tunnel: w197 -> [_ w318]
      frame False {
      }
      frame True {
        n154 = for {
          tunnel: w333 -> [w396] mode=indexing
          tunnel: w332 -> [w401] mode=indexing
          shift-right: [w397] -> w330
          shift-left: waveform(dbl)[] [] -> [w398]
          shift-right: [w394] -> w324
          shift-left: string[] [] -> [w391]
          n155 = Less?(x=w401, y=13.0) -> (x < y?=w399:bool)
          n156 = case shown="True" w399 {
            tunnel: w396 -> [_ w405]
            tunnel: [w402 w404] -> w397
            tunnel: w398 -> [w402 w403]
            frame False {
            }
            frame True {
              n157 = Build Array (concatenate)(w405, w403) -> (w404:waveform(dbl)[])
            }
          }
          n158 = Get Waveform Attribute(6:"NI_ChannelName" ("name"), 7:w396) -> (1:w393:variant)  [unwired: 2 in, 3 out]
          n159 = Variant To Flattened String(Variant=w393) -> (data string=w392:string)  [unwired: 1 out]
          n160 = Build Array (concatenate)(w392, w391) -> (w394:string[])
        }
        n161 = Obtain Queue(name (unnamed)="Downsampled", element data type=waveform(dbl)[] [], create if not found? (T)=FALSE) -> (queue out=w319:refnum<queue>)  [unwired: 2 in, 2 out]
        n162 = case shown="\"IV Monitor\"" w318 {
          tunnel: w330 -> [w337 w340]
          tunnel: w328 -> [_ w339]
          tunnel: [w337 w341] -> w323
          tunnel: w319 -> [w338 w342]
          frame "RT Monitor", Default {
            n163 = call "DownSampleData_MaxMin.vi"("Desired Sampling Rate"=500.0, "Oversampled Values"=w337) -> ("Downsampled Data"=w336:waveform(sgl)[])  [unwired: 8 in, 1 out]
            n164 = Enqueue Element(queue=w338, element=w336, timeout in ms (-1)=25) -> ()  [unwired: 1 in, 3 out]
          }
          frame "IV Monitor" {
            n165 = Build Array (concatenate)(w339, w340) -> (w341:waveform(dbl)[])
            n166 = call "DownSampleData_82.vi"("Desired Sampling Rate"=500.0, "Oversampled Values"=w341) -> ("Downsampled Data"=w345:waveform(sgl)[])  [unwired: 8 in, 1 out]
            n167 = Enqueue Element(queue=w342, element=w345, timeout in ms (-1)=25) -> ()  [unwired: 1 in, 3 out]
          }
        }
        n168 = local read "tdms file out"() -> (w326:refnum<k34>)
        n169 = local read "FileOpen"() -> (w327:bool)
        n170 = case shown="True" w327 {
          tunnel: w326 -> [_ w351]
          tunnel: enum16{"decimated", "interleaved"}."decimated" ("data layout (0:decimated)") -> [_ w350]
          tunnel: w324 -> [_ w349]
          tunnel: w323 -> [_ w348]
          tunnel: w318 -> [_ w346]
          frame False {
          }
          frame True {
            n171 = flat-sequence {
              tunnel: w351 -> [w357]
              tunnel: w350 -> [w356]
              tunnel: w349 -> [w355]
              tunnel: w348 -> [w354]
              tunnel: [w352] -> w347
              tunnel: w347 -> [w359]
              tunnel: w346 -> [w358]
              frame #0 {
                n172 = TDMS Write(0:w357, 1:w356, 7:w355, 9:w354) -> (4:w352:refnum<k34>, 15:w353:errorcluster)  [unwired: 2 in, 2 out]
                n173 = local write "error out"(w353) -> ()
              }
              frame #1 {
                n174 = local read "fileCreateTime"() -> (w363:timestamp)
                n175 = Get Date/Time In Seconds() -> (seconds since 1Jan1904=w362:timestamp)
                n176 = Subtract(x=w362, y=w363) -> (x-y=w364:dbl)
                n177 = Greater?(x=w364, y=30.0) -> (0:w360:bool)
                n178 = case shown="True" w360 {
                  tunnel: w359 -> [_ w367]
                  tunnel: w358 -> [_ w366]
                  frame False {
                  }
                  frame True {
                    n179 = TDMS Close(11:w367) -> ()  [unwired: 1 in, 2 out]
                    n180 = local read "output path"() -> (w378:path)
                    n181 = call <vilib>:"Check if File or Folder Exists.vi"("path"=w378) -> ("file or folder exists?"=w387:bool, "dup path"=w382:path)  [unwired: 8 in, 1 out]
                    n182 = Get Date/Time In Seconds() -> (seconds since 1Jan1904=w368:timestamp)
                    n183 = local read "Analyte"() -> (w371:string)
                    n184 = local write "fileCreateTime"(w368) -> ()
                    n185 = Format Date/Time String(time format string (%c)="%y%m%d_%H%M%S_", seconds (now)=w368) -> (date/time string=w377:string)  [unwired: 1 in]
                    n186 = case shown="False" w387 {
                      tunnel: w382 -> [w389 w390]
                      tunnel: [w388 w390] -> w383
                      frame False {
                        n187 = Create Folder(path (use dialog)=w389) -> (created path=w388:path)  [unwired: 2 in, 2 out]
                      }
                      frame True {
                      }
                    }
                    n188 = local read "ParameterNames"() -> (w375:string[])
                    n189 = Concatenate Strings(w377, w371, ".tdms" ("string")) -> (w376:string)
                    n190 = local read "ParameterValues"() -> (w370:string[])
                    n191 = Build Path(base path=w383, name or relative path=w376) -> (appended path=w381:path)
                    n192 = Format Into String(w366) -> (resulting string=w365:string)  [unwired: 3 in, 1 out]
                    n193 = Build Array (concatenate)(w375, "mode") -> (w372:string[])
                    n194 = Build Array (concatenate)(w370, w365) -> (w373:string[])
                    n195 = TDMS Open(5:FALSE ("create index file? (T)"), 10:T3."create" ("operation (0:open)"), 11:w381) -> (3:w386:refnum<k34>)  [unwired: 4 in, 1 out]
                    n196 = TDMS Set Properties(5:w373, 7:w372, 11:w386) -> (3:w369:refnum<k34>)  [unwired: 3 in, 3 out]
                    n197 = local write "tdms file out"(w369) -> ()
                  }
                }
              }
            }
          }
        }
      }
    }
    n198 = local read "StopProgram"() -> (w205:bool)
  }
  n199 = while {
    tunnel: w17 -> [w413]
    tunnel: w15 -> [w411]
    stop <- w414 stop-if-true
    n200 = Dequeue Element(queue=w413) -> (element=w412:cluster{"Command":string})  [unwired: 2 in, 3 out]
    n201 = Unbundle By Name(w412) -> ("Command"=w410:string)
    n202 = case shown="\"RT_Curve\"" w410 {
      tunnel: w411 -> [_ w478 _ _ _ w657 _]
      frame "RT_Curve" {
        n203 = local write "Recording"(TRUE ("Recording")) -> ()
        n204 = property on="Record" class="Bool (strict)"("BoolText.Text"="Stop" ("Boolean Text.Text")) -> ()  [unwired: 2 in, 2 out]
        n205 = Get Date/Time In Seconds() -> (seconds since 1Jan1904=w415:timestamp)
        n206 = local read "Analyte"() -> (w421:string)
        n207 = local write "fileCreateTime"(w415) -> ()
        n208 = Format Date/Time String(time format string (%c)="%y%m%d_%H%M%S_", seconds (now)=w415) -> (date/time string=w422:string)  [unwired: 1 in]
        n209 = local read "FilenameValid"() -> (w425:bool)
        n210 = Concatenate Strings(w422, w421, "RT.tdms" ("string")) -> (w420:string)
        n211 = Obtain Queue(name (unnamed)="InternalCommands", element data type=cluster{"Command":string} {"Command"=""}, create if not found? (T)=FALSE) -> (queue out=w416:refnum<queue>)  [unwired: 2 in, 2 out]
        n212 = case shown="True" w425 {
          tunnel: w420 -> [_ w438]
          tunnel: w416 -> [w428 _]
          frame False {
            n213 = property on="Record" class="Bool (strict)"("BoolText.Text"="Record" ("Boolean Text.Text")) -> ()  [unwired: 2 in, 2 out]
            n214 = Lossy Enqueue Element(queue=w428, element=cluster{"Command":string} {"Command"="MonitorClose"}) -> ()  [unwired: 1 in, 4 out]
            n215 = local write "Warnings"("Wafer, Chip and Analyte must be filled" ("Warnings")) -> ()
          }
          frame True {
            w436 = enum32{"RT Monitor", "IV Monitor"}."RT Monitor" ("Tab Control 2")
            n216 = local read "output path"() -> (w439:path)
            n217 = call <vilib>:"Check if File or Folder Exists.vi"("path"=w439) -> ("file or folder exists?"=w448:bool, "dup path"=w442:path)  [unwired: 8 in, 1 out]
            n218 = case shown="False" w448 {
              tunnel: w442 -> [w471 w472]
              tunnel: [w470 w472] -> w444
              frame False {
                n219 = Create Folder(path (use dialog)=w471) -> (created path=w470:path)  [unwired: 2 in, 2 out]
              }
              frame True {
              }
            }
            n220 = local read "ParameterNames"() -> (w441:string[])
            n221 = local read "ParameterValues"() -> (w440:string[])
            n222 = Build Path(base path=w444, name or relative path=w438) -> (appended path=w443:path)
            n223 = property on="Tab Control 2" class="TabCtl (strict)"("Value"=w436) -> ()  [unwired: 2 in, 2 out]
            n224 = Format Into String(w436) -> (resulting string=w434:string)  [unwired: 3 in, 1 out]
            n225 = Build Array (concatenate)(w441, "Mode") -> (w433:string[])
            n226 = Build Array (concatenate)(w440, w434) -> (w435:string[])
            n227 = TDMS Open(5:FALSE ("create index file? (T)"), 10:T3."create" ("operation (0:open)"), 11:w443) -> (3:w447:refnum<k34>)  [unwired: 4 in, 1 out]
            n228 = TDMS Set Properties(5:w435, 7:w433, 11:w447) -> (3:w449:refnum<k34>)  [unwired: 3 in, 3 out]
            n229 = flat-sequence {
              tunnel: w449 -> [w452]
              tunnel: ["TraceTime"] -> w437
              tunnel: w437 -> [w455]
              frame #0 {
                n230 = local write "Means"(dbl[] [] ("Means")) -> ()
                n231 = local write "stds"(dbl[] [] ("stds")) -> ()
                "tdms file out" <- w452
              }
              frame #1 {
                n232 = local write "FileOpen"(TRUE ("FileOpen")) -> ()
              }
              frame #2 {
                w456 = cluster{"Command":string, "Time":i32} {"Command"="", "Time"=0}
                n233 = call <vilib>:"High Resolution Relative Seconds.vi"() -> ("relative seconds"=w467:dbl)
                n234 = Add(x=w467, y=w455) -> (x+y=w463:dbl)
                n235 = Add(x=w463, y=0.5) -> (x+y=w462:dbl)
                n236 = Bundle By Name(cluster=w456, "Command"="MonitorClose", "Time"=w463) -> (w469:cluster{"Command":string, "Time":i32})
                n237 = Obtain Queue(name (unnamed)="DelayTime", element data type=cluster{"Command":string, "Time":i32} {"Command"="", "Time"=0}, create if not found? (T)=FALSE) -> (queue out=w457:refnum<queue>)  [unwired: 2 in, 2 out]
                n238 = Bundle By Name(cluster=w456, "Command"="FileClose", "Time"=w462) -> (w466:cluster{"Command":string, "Time":i32})
                n239 = Enqueue Element(queue=w457, element=w469) -> (queue out=w461:refnum<queue>)  [unwired: 2 in, 2 out]
                n240 = Enqueue Element(queue=w461, element=w466) -> ()  [unwired: 2 in, 3 out]
              }
            }
          }
        }
      }
      frame "MonitorOpen" {
        n241 = flat-sequence {
          tunnel: w478 -> [w481]
          tunnel: [w481] -> w477
          tunnel: w477 -> [w483]
          tunnel: w473 -> [w486]
          frame #0 {
            n242 = local write "FileOpen"(FALSE ("FileOpen")) -> ()
          }
          frame #1 {
            w485 = 10123 items=["Finite Samples"=10178, "Continuous Samples"=10123, "Hardware Timed Single Point"=12522] ("sample mode")
            n243 = call <vilib>:"DAQmx Stop Task.vi"("task/channels in"=w483) -> ("task out"=w482:refnum<k21>)  [unwired: 13 in, 1 out]
            n244 = local read "Sampling Rate:"() -> (w484:dbl)
            n245 = call-poly <vilib>:"DAQmx Timing.vi"("task/channels in"=w482, "sample mode"=w485, "rate"=w484) -> ()  [unwired: 11 in, 2 out]
          }
          frame #2 {
            n246 = Lossy Enqueue Element(queue=w486, element=cluster{"Command":string} {"Command"="Monitor"}) -> ()  [unwired: 1 in, 4 out]
          }
        }
        n247 = local write "Monitoring"(TRUE ("Monitoring")) -> ()
        n248 = Obtain Queue(name (unnamed)="InternalCommands", element data type=cluster{"Command":string} {"Command"=""}, create if not found? (T)=FALSE) -> (queue out=w473:refnum<queue>)  [unwired: 2 in, 2 out]
      }
      frame "IV_Curve" {
        n249 = local read "FilenameValid"() -> (w488:bool)
        n250 = case shown="True" w488 {
          frame False {
            n251 = Obtain Queue(name (unnamed)="InternalCommands", element data type=cluster{"Command":string} {"Command"=""}, create if not found? (T)=FALSE) -> (queue out=w489:refnum<queue>)  [unwired: 2 in, 2 out]
            n252 = Lossy Enqueue Element(queue=w489, element=cluster{"Command":string} {"Command"="MonitorClose"}) -> ()  [unwired: 1 in, 4 out]
          }
          frame True {
            w513 = enum32{"RT Monitor", "IV Monitor"}."IV Monitor" ("Tab Control 2")
            n253 = local read "output path"() -> (w523:path)
            n254 = call <vilib>:"Check if File or Folder Exists.vi"("path"=w523) -> ("file or folder exists?"=w537:bool, "dup path"=w531:path)  [unwired: 8 in, 1 out]
            n255 = Get Date/Time In Seconds() -> (seconds since 1Jan1904=w514:timestamp)
            "fileCreateTime" <- w514
            n256 = local read "Analyte"() -> (w521:string)
            n257 = case shown="False" w537 {
              tunnel: w531 -> [w631 w632]
              tunnel: [w630 w632] -> w532
              frame False {
                n258 = Create Folder(path (use dialog)=w631) -> (created path=w630:path)  [unwired: 2 in, 2 out]
              }
              frame True {
              }
            }
            n259 = Format Date/Time String(time format string (%c)="%y%m%d_%H%M%S_", seconds (now)=w514) -> (date/time string=w522:string)  [unwired: 1 in]
            n260 = local read "ParameterNames"() -> (w519:string[])
            n261 = Concatenate Strings(w522, w521, "IV.tdms" ("string")) -> (w520:string)
            n262 = Build Path(base path=w532, name or relative path=w520) -> (appended path=w530:path)
            n263 = local read "ParameterValues"() -> (w518:string[])
            n264 = property on="Tab Control 2" class="TabCtl (strict)"("Value"=w513) -> ()  [unwired: 2 in, 2 out]
            n265 = Format Into String(w513) -> (resulting string=w512:string)  [unwired: 3 in, 1 out]
            n266 = Build Array (concatenate)(w519, "mode") -> (w515:string[])
            n267 = Build Array (concatenate)(w518, w512) -> (w516:string[])
            n268 = TDMS Open(5:FALSE ("create index file? (T)"), 10:T3."create" ("operation (0:open)"), 11:w530) -> (3:w536:refnum<k34>)  [unwired: 4 in, 1 out]
            n269 = TDMS Set Properties(5:w516, 7:w515, 11:w536) -> (3:w533:refnum<k34>)  [unwired: 3 in, 3 out]
            n270 = flat-sequence {
              tunnel: w533 -> [w540]
              tunnel: [w552] -> w527
              tunnel: [w558] -> w526
              tunnel: [w553] -> w510
              tunnel: [w551] -> w507
              tunnel: [w545] -> w506
              tunnel: [w542] -> w501
              tunnel: [w550] -> w499
              tunnel: [w546] -> w494
              tunnel: [w576] -> w528
              tunnel: w527 -> [w578]
              tunnel: w526 -> [w579]
              tunnel: [w580] -> w511
              tunnel: w510 -> [w580]
              tunnel: [w575] -> w508
              tunnel: w507 -> [w575]
              tunnel: w506 -> [w574]
              tunnel: [w574] -> w505
              tunnel: [w573] -> w502
              tunnel: w501 -> [w573]
              tunnel: w499 -> [w572]
              tunnel: [w572] -> w498
              tunnel: [w571] -> w495
              tunnel: w494 -> [w571]
              tunnel: [w601] -> w529
              tunnel: w528 -> [w601]
              tunnel: w511 -> [w587]
              tunnel: [w586] -> w509
              tunnel: w508 -> [w586]
              tunnel: w505 -> [w585]
              tunnel: [w585] -> w504
              tunnel: [w584] -> w503
              tunnel: w502 -> [w584]
              tunnel: [w583] -> w500
              tunnel: w498 -> [w582]
              tunnel: [w582] -> w497
              tunnel: [w581] -> w496
              tunnel: w495 -> [w581]
              tunnel: w529 -> [w608]
              tunnel: w509 -> [w611]
              tunnel: w504 -> [w610]
              tunnel: w503 -> [w609]
              tunnel: w500 -> [w607]
              tunnel: w497 -> [w605]
              tunnel: w496 -> [w602]
              frame #0 {
                n271 = local write "tdms file out"(w540) -> ()
                n272 = local write "stds"(dbl[] [] ("stds")) -> ()
                n273 = local write "Means"(dbl[] [] ("Means")) -> ()
              }
              frame #1 {
                w548 = 5000.0 ("#s")
                w551 = T7."Triangle Wave" ("signal type")
                w566 = 10123 items=["Finite Samples"=10178, "Continuous Samples"=10123, "Hardware Timed Single Point"=12522] ("sample mode")
                w562 = -1 items=["Default"=-1, "RSE"=10083, "Differential"=10106, "Pseudodifferential"=12529] ("output terminal configuration")
                n274 = local write "FileOpen"(TRUE ("FileOpen")) -> ()
                n275 = call <vilib>:"DAQmx Create Task.vi"("auto cleanup"=TRUE) -> ("task out"=w568:refnum<k21>, "error out"=w567:errorcluster)  [unwired: 13 in]
                n276 = call-poly <vilib>:"DAQmx Create Virtual Channel.vi"("task in"=w568, "maximum value"=10.0, "minimum value"=-10.0, "output terminal configuration"=w562, "physical channels"=tag "Dev1/ao0", "error in"=w567) -> ("task out"=w569:refnum<k21>)  [unwired: 8 in, 1 out]
                n277 = local read "Bias Voltage (mV)"() -> (w544:string)
                n278 = call-poly <vilib>:"DAQmx Timing.vi"("task/channels in"=w569, "sample mode"=w566, "samples per channel"=2560, "rate"=2500.0) -> ("task out"=w559:refnum<k21>)  [unwired: 10 in, 1 out]
                n279 = property class="DAQmx Timing"(reference=w559) -> (reference out=w558:refnum<k21>, "SampClk.Rate"=w547:dbl)  [unwired: 1 in, 1 out]
                n280 = Decimal String To Number(string=w544) -> (number=w543:i32)  [unwired: 2 in, 1 out]
                n281 = Divide(x=w548, y=w547) -> (x/y=w546:dbl)
                n282 = local read "frequency"() -> (w545:dbl)
                n283 = Divide(x=w543, y=1000) -> (x/y=w542:dbl)
                n284 = Bundle By Name(cluster=cluster{"Fs":dbl, "#s":dbl} {"Fs"=1000.0, "#s"=1000.0} ("sampling info"), "#s"=w548, "Fs"=w547) -> (w550:cluster{"Fs":dbl, "#s":dbl})
                n285 = call <vilib>:"Basic Function Generator.vi"("reset signal"=TRUE, "sampling info"=w550, "signal type"=w551, "phase"=0.0, "amplitude"=w542, "frequency"=w545) -> ("signal out"=w557:waveform(dbl))  [unwired: 3 in, 2 out]
                n286 = local read "TraceTime"() -> (w553:dbl)
                n287 = Build Array(w557) -> (w552:waveform(dbl)[])
              }
              frame #2 {
                (unwired) TRUE ("auto start")
                n288 = call-poly <vilib>:"DAQmx Write.vi"("task/channels in"=w579, "data"=w578) -> ("task out"=w577:refnum<k21>)  [unwired: 11 in, 2 out]
                n289 = call <vilib>:"DAQmx Start Task.vi"("task/channels in"=w577) -> ("task out"=w576:refnum<k21>)  [unwired: 13 in, 1 out]
              }
              frame #3 {
                w588 = cluster{"Command":string, "Time":i32} {"Command"="", "Time"=0}
                n290 = call <vilib>:"High Resolution Relative Seconds.vi"() -> ("relative seconds"=w598:dbl)
                n291 = Add(x=w598, y=w587) -> (x+y=w583:dbl)
                n292 = Add(x=w583, y=0.0) -> (x+y=w594:dbl)
                n293 = Bundle By Name(cluster=w588, "Command"="MonitorClose", "Time"=w583) -> (w600:cluster{"Command":string, "Time":i32})
                n294 = Obtain Queue(name (unnamed)="DelayTime", element data type=cluster{"Command":string, "Time":i32} {"Command"="", "Time"=0}, create if not found? (T)=FALSE) -> (queue out=w589:refnum<queue>)  [unwired: 2 in, 2 out]
                n295 = Bundle By Name(cluster=w588, "Command"="FileClose", "Time"=w594) -> (w597:cluster{"Command":string, "Time":i32})
                n296 = Enqueue Element(queue=w589, element=w600) -> (queue out=w593:refnum<queue>)  [unwired: 2 in, 2 out]
                n297 = Enqueue Element(queue=w593, element=w597) -> ()  [unwired: 2 in, 3 out]
              }
              frame #4 {
                n298 = node-c288(w602) -> (w604:T4)  [unwired: 3 in]
                n299 = timed-loop {
                  tunnel: w611 -> [w623]
                  tunnel: w610 -> [w622]
                  tunnel: w609 -> [w621]
                  tunnel: w608 -> [w618]
                  tunnel: w607 -> [w616]
                  tunnel: [w614] -> w606
                  tunnel: w605 -> [w613]
                  timing: w604 -> [_]
                  timing-out: [_] -> w603
                  stop <- w615 stop-if-true
                  n300 = node-c288() -> ()  [unwired: 1 in, 1 out]
                  n301 = call <vilib>:"Basic Function Generator.vi"("sampling info"=w613, "signal type"=w623, "amplitude"=w621, "frequency"=w622) -> ("signal out"=w620:waveform(dbl))  [unwired: 5 in, 2 out]
                  n302 = call <vilib>:"High Resolution Relative Seconds.vi"() -> ("relative seconds"=w617:dbl)
                  n303 = Greater?(x=w617, y=w616) -> (0:w615:bool)
                  n304 = Build Array(w620) -> (w619:waveform(dbl)[])
                  n305 = call-poly <vilib>:"DAQmx Write.vi"("task/channels in"=w618, "data"=w619) -> ("task out"=w614:refnum<k21>)  [unwired: 11 in, 2 out]
                  n306 = node-c288() -> ()  [unwired: 1 in, 1 out]
                }
                n307 = node-c288(w603) -> ()  [unwired: 1 out]
                n308 = call <vilib>:"DAQmx Stop Task.vi"("task/channels in"=w606) -> ("task out"=w612:refnum<k21>)  [unwired: 13 in, 1 out]
                n309 = call <vilib>:"DAQmx Clear Task.vi"("task in"=w612) -> ()  [unwired: 14 in, 1 out]
              }
            }
          }
        }
      }
      frame Default {
      }
      frame "ParameterRead" {
        w645 = "" ("y")
        n310 = local read "Wafer, Chip"() -> (w643:string)
        n311 = local read "Analyte"() -> (w639:string)
        n312 = local read "Reference Voltage (mV)"() -> (w647:string)
        n313 = Not Equal?(x=w643, y=w645) -> (x != y?=w634:bool)
        n314 = Not Equal?(x=w639, y=w645) -> (x != y?=w636:bool)
        n315 = local read "Experiment Name"() -> (w650:string)
        n316 = local read "Bias Voltage (mV)"() -> (w648:string)
        n317 = call <vilib>:"Delimited String to 1D String Array.vi"("delimiter"="," ("search string/char (-)"), "delimited string"=w643) -> ("string array"=w641:string[])  [unwired: 9 in]
        n318 = local read "DataDirectory"() -> (w646:path)
        n319 = Or(x=w636, y=w634) -> (x .or. y?=→"FilenameValid":bool)
        n320 = Index Array(array=w641) -> (element #1=w640:string, element #2=w638:string)  [unwired: 2 in]
        n321 = local read "Notes"() -> (w651:string)
        n322 = local read "Buffer"() -> (w649:string)
        n323 = Build Path(base path=w646, name or relative path=w640) -> (appended path=w637:path)
        n324 = Build Array(w640, w651, w650, w649, w648, w647, w638, w639) -> (→"ParameterValues":string[])
        n325 = Build Path(base path=w637, name or relative path=w638) -> (appended path=→"output path":path)
        "ParameterNames" <- string[] ["Wafer", "Notes", "Experiment Name", "Buffer", "Bias Voltage", "Reference Electrode", "Chip", "Analyte"]
      }
      frame "MonitorClose" {
        n326 = local write "Monitoring"(FALSE ("Monitoring")) -> ()
        n327 = flat-sequence {
          tunnel: w657 -> [w659]
          tunnel: w653 -> [w660]
          frame #0 {
            n328 = call <vilib>:"DAQmx Stop Task.vi"("task/channels in"=w659) -> ()  [unwired: 13 in, 2 out]
          }
          frame #1 {
            n329 = Lossy Enqueue Element(queue=w660, element=cluster{"Command":string} {"Command"="Close"}) -> ()  [unwired: 1 in, 4 out]
          }
        }
        n330 = Obtain Queue(name (unnamed)="InternalCommands", element data type=cluster{"Command":string} {"Command"=""}, create if not found? (T)=FALSE) -> (queue out=w653:refnum<queue>)  [unwired: 2 in, 2 out]
      }
      frame "FileClose" {
        n331 = flat-sequence {
          frame #0 {
            w662 = FALSE ("RT Monitoring")
            n332 = local write "FileOpen"(FALSE ("FileOpen")) -> ()
            n333 = property on="Record" class="Bool (strict)"("Value"=FALSE ("Record")) -> ()  [unwired: 2 in, 2 out]
            n334 = property on="Record" class="Bool (strict)"("BoolText.Text"="Record" ("Boolean Text.Text")) -> ()  [unwired: 2 in, 2 out]
            n335 = property on="RT Monitoring" class="Bool (strict)"("Value"=w662) -> ()  [unwired: 2 in, 2 out]
            n336 = property on="IV Monitoring" class="Bool (strict)"("Value"=w662) -> ()  [unwired: 2 in, 2 out]
            n337 = local write "Warnings"("File has been saved" ("Warnings")) -> ()
          }
          frame #1 {
          }
          frame #2 {
            n338 = local write "Recording"(FALSE ("Recording")) -> ()
          }
          frame #3 {
            n339 = local read "tdms file out"() -> (w668:refnum<k34>)
            n340 = TDMS Close(11:w668) -> (0:w669:errorcluster)  [unwired: 1 in, 1 out]
            n341 = local write "error out"(w669) -> ()
          }
        }
      }
    }
    n342 = local read "StopProgram"() -> (w414:bool)
  }
  n343 = while {
    tunnel: w12 -> [w694]
    tunnel: [w694] -> w11
    tunnel: w8 -> [w691]
    tunnel: w6 -> [w673]
    tunnel: [w672] -> w5
    stop <- w695 stop-if-true
    n344 = Get Queue Status(queue=w694) -> (queue out=w677:refnum<queue>, # elements in queue=→"# elements in queue":i32)  [unwired: 2 in, 6 out]
    n345 = Dequeue Element(queue=w677) -> (element=w678:waveform(dbl)[], timed out?=→"timed out?":bool)  [unwired: 2 in, 2 out]
    n346 = Concatenate Strings(w691, "GetTraceResult" ("string")) -> (w682:string)
    n347 = for {
      tunnel: w678 -> [w708] mode=indexing
      tunnel: [w709] -> w698
      tunnel: [w705] -> w697 mode=indexing
      n348 = Unbundle By Name(w708) -> ("dt"=w709:dbl)
      n349 = Get Waveform Attribute(6:"NI_ChannelName" ("name"), 7:w708) -> (1:w706:variant)  [unwired: 2 in, 3 out]
      n350 = Variant To Data(type="", Variant=w706) -> (data=w705:string)  [unwired: 1 in, 1 out]
    }
    n351 = call <vilib>:"AddHeader.vi"("client handle"=w673, "header"="Content-Type", "value"="application/json") -> ("client handle out"=w683:T2)  [unwired: 11 in, 1 out]
    n352 = for {
      tunnel: w678 -> [w703] mode=indexing
      tunnel: [w701] -> w696 mode=indexing
      n353 = Unbundle By Name(w703) -> ("Y"=w702:dbl[])
      n354 = To Single Precision Float(number=w702) -> (single precision float=w701:sgl[])
    }
    n355 = property on="Tab Control 2" class="TabCtl (strict)"() -> ("Value"=w680:enum32{"RT Monitor", "IV Monitor"})  [unwired: 2 in, 2 out]
    n356 = Format Into String(w680) -> (resulting string=w679:string)  [unwired: 3 in, 1 out]
    n357 = local read "Means"() -> (w671:dbl[])
    n358 = local read "stds"() -> (w670:dbl[])
    n359 = Bundle By Name(cluster=T8 {"channelNames"=[], "dt"=0.0, "traces"=[], "dataType"="", "means"=[], "stds"=[]}, "dt"=w698, "channelNames"=w697, "traces"=w696, "dataType"=w679, "means"=w671, "stds"=w670) -> (w699:T8)
    n360 = Flatten To JSON(anything=w699) -> (JSON string=w689:string)  [unwired: 2 in, 1 out]
    n361 = Bundle By Name(cluster=cluster{"data":string, "dataType":string} {"data"="", "dataType"=""}, "data"=w689, "dataType"=w679) -> (w688:cluster{"data":string, "dataType":string})
    n362 = Flatten To JSON(anything=w688) -> (JSON string=w687:string)  [unwired: 2 in, 1 out]
    n363 = call-poly <vilib>:"POST.vi"("client handle"=w683, "url"=w682, "buffer"=w687, "timeout (10000)"=10000) -> ("client handle out"=w672:T2, "headers"=→"headers":string, "body"=→"body 2":string, "error out"=→"error out 3":errorcluster)  [unwired: 8 in]
    n364 = local read "StopProgram"() -> (w695:bool)
  }
  n365 = while {
    tunnel: w13 -> [w721]
    tunnel: [w718] -> w10
    tunnel: w9 -> [w717]
    tunnel: w3 -> [w712]
    tunnel: [w711] -> w2
    tunnel: w1 -> [w710]
    stop <- w726 stop-if-true
    n366 = while {
      tunnel: [w804] -> w722
      tunnel: w717 -> [w800]
      tunnel: w712 -> [w799]
      tunnel: [w798] -> w711
      stop <- w801 stop-if-true
      n367 = call <vilib>:"GET.vi"("client handle"=w799, "url"=w800, "timeout (10000)"=60000) -> ("client handle out"=w798:T2, "body"=w804:string, "error out"=w803:errorcluster)  [unwired: 9 in, 1 out]
      "error out 2" <- w803
      n368 = Unbundle By Name(w803) -> ("status"=w802:bool)
      n369 = Not(x=w802) -> (.not. x?=w801:bool)
    }
    "body" <- w722
    n370 = Unflatten From JSON(JSON string=w722, type and defaults=w721) -> (value=w720:T1, error out=w715:errorcluster)  [unwired: 5 in]
    n371 = local write "error out"(w715) -> ()
    n372 = Unbundle By Name(w720) -> ("command"=w716:string, "payload"=w719:string)
    n373 = Obtain Queue(name (unnamed)="UserCommands", element data type=cluster{"Command":string} {"Command"=""}, create if not found? (T)=FALSE) -> (queue out=w718:refnum<queue>)  [unwired: 2 in, 2 out]
    n374 = flat-sequence {
      tunnel: w719 -> [w731]
      tunnel: w718 -> [w730]
      tunnel: w716 -> [w729]
      tunnel: [w728] -> w714
      tunnel: [w727] -> w713
      tunnel: w714 -> [w797]
      tunnel: w713 -> [w790]
      tunnel: w710 -> [w789]
      frame #0 {
        n375 = case shown="\"StartIV\", \"StartRT\"" w729 {
          tunnel: w730 -> [_ w742 w758]
          tunnel: w731 -> [_ w740 w759]
          tunnel: w729 -> [_ w737 w756]
          tunnel: ["NoCommand" ("source") w734 w757] -> w728
          tunnel: ["error" ("command") w736 w755] -> w727
          frame "False", Default {
          }
          frame "LBParameters" {
            n376 = Unflatten From JSON(JSON string=w740, type and defaults=T9 {"channels"="", "analyte"="", "notes"="", "buffer"="", "experiment"="", "waferChip"=""}) -> (value=w739:T9, error out=w738:errorcluster)  [unwired: 5 in]
            n377 = flat-sequence {
              tunnel: w739 -> [w752]
              tunnel: w742 -> [w754]
              frame #0 {
                n378 = Unbundle By Name(w752) -> ("channels"=w751:string, "analyte"=w750:string, "notes"=w749:string, "buffer"=w748:string, "experiment"=w747:string, "waferChip"=w746:string)
                n379 = local write "Notes"(w749) -> ()
                n380 = local write "Buffer"(w748) -> ()
                n381 = local write "Analyte"(w750) -> ()
                n382 = local write "Experiment Name"(w747) -> ()
                n383 = local write "Wafer, Chip"(w746) -> ()
                n384 = local write "Channels"(w751) -> ()
              }
              frame #1 {
                n385 = Enqueue Element(queue=w754, element=cluster{"Command":string} {"Command"="ParameterRead"}) -> ()  [unwired: 2 in, 3 out]
              }
            }
            n386 = Unbundle By Name(w738) -> ("source"=w735:string)
            n387 = case shown="No Error" w738 {
              tunnel: w737 -> [w743 _]
              tunnel: [w743 "error" ("command")] -> w736
              tunnel: w735 -> [_ w744]
              tunnel: [w743 w744] -> w734
              frame No Error {
              }
              frame Error {
              }
            }
          }
          frame "StartIV", "StartRT" {
            n388 = flat-sequence {
              tunnel: w759 -> [w770]
              tunnel: [w761] -> w757
              tunnel: w756 -> [w764]
              tunnel: [w763] -> w755
              tunnel: w756 -> [w776]
              tunnel: w758 -> [w775]
              frame #0 {
                n389 = Unflatten From JSON(JSON string=w770, type and defaults=T10 {"duration"=0.0, "bias"=0.0, "frequency"=0.0}) -> (value=w769:T10, error out=w765:errorcluster)  [unwired: 5 in]
                n390 = Unbundle By Name(w769) -> ("duration"=w767:dbl, "bias"=w768:dbl, "frequency"=→"frequency":dbl)
                n391 = Unbundle By Name(w765) -> ("source"=w762:string)
                n392 = local write "TraceTime"(w767) -> ()
                n393 = case shown="No Error" w765 {
                  tunnel: w764 -> [w772 _]
                  tunnel: [w772 "error" ("command")] -> w763
                  tunnel: w762 -> [_ w773]
                  tunnel: [w772 w773] -> w761
                  frame No Error {
                  }
                  frame Error {
                  }
                }
                n394 = Number To Decimal String(number=w768) -> (decimal integer string=w766:string)  [unwired: 1 in]
                n395 = local write "Bias Voltage (mV)"(w766) -> ()
              }
              frame #1 {
                n396 = case shown="\"StartRT\", Default" w776 {
                  tunnel: w775 -> [w777 w788]
                  frame "StartRT", Default {
                    n397 = Enqueue Element(queue=w777, element=cluster{"Command":string} {"Command"="ParameterRead"}) -> (queue out=w778:refnum<queue>)  [unwired: 2 in, 2 out]
                    n398 = Enqueue Element(queue=w778, element=cluster{"Command":string} {"Command"="MonitorOpen"}) -> (queue out=w780:refnum<queue>)  [unwired: 2 in, 2 out]
                    n399 = Lossy Enqueue Element(queue=w780, element=cluster{"Command":string} {"Command"="RT_Curve"}) -> ()  [unwired: 1 in, 4 out]
                  }
                  frame "StartIV" {
                    n400 = Enqueue Element(queue=w788, element=cluster{"Command":string} {"Command"="ParameterRead"}) -> (queue out=w783:refnum<queue>)  [unwired: 2 in, 2 out]
                    n401 = Enqueue Element(queue=w783, element=cluster{"Command":string} {"Command"="MonitorOpen"}) -> (queue out=w785:refnum<queue>)  [unwired: 2 in, 2 out]
                    n402 = Lossy Enqueue Element(queue=w785, element=cluster{"Command":string} {"Command"="IV_Curve"}) -> ()  [unwired: 1 in, 4 out]
                  }
                }
              }
            }
          }
        }
      }
      frame #1 {
        n403 = Concatenate Strings(w789, w790, "&message=" ("string"), w797) -> (w792:string)
        n404 = call <vilib>:"Escape HTTP URL.vi"("unescaped string in"=w792) -> ("escaped string out"=w791:string)
        n405 = call <vilib>:"OpenHandle.vi"("verify server(true)"=FALSE) -> ("client handle out"=w795:T2)  [unwired: 13 in, 1 out]
        n406 = call <vilib>:"GET.vi"("client handle"=w795, "url"=w791) -> ("client handle out"=w794:T2)  [unwired: 10 in, 3 out]
        n407 = call <vilib>:"CloseHandle.vi"("client handle"=w794) -> ()  [unwired: 14 in, 1 out]
      }
    }
    n408 = local read "StopProgram"() -> (w726:bool)
  }
  n409 = Release Queue(queue=w11) -> ()  [unwired: 2 in, 3 out]
  n410 = call <vilib>:"CloseHandle.vi"("client handle"=w5) -> ()  [unwired: 14 in, 1 out]
  n411 = call <vilib>:"CloseHandle.vi"("client handle"=w2) -> ()  [unwired: 14 in, 1 out]
  n412 = Release Queue(queue=w10) -> ()  [unwired: 2 in, 3 out]
